vi "CRYCalibration Editor.vi"() -> ()   [LabVIEW 2013]
uses:
  <vilib>/Utility/miscctls.llb/LVBoundsTypeDef.ctl
  Typedef Control/CRYCalibration All Cluster.ctl
  Typedef Control/CRYCalibration 2DCluster.ctl
  Typedef Control/CRYCalibration Cluster.ctl
  Typedef Control/CRYData Cluster.ctl
  CRYProject/CRYProject Editor Global.vi
  CRYMainGlobal.vi
  CRYWindow/SubVI/CRYMain Sub Window Global.vi
  SubVI/CRYCal Global.vi
  Misc/SubVI/CRYMisc vis settings global.vi
panel:
  out "Signal Type Index":i32
  out "Origine Calibration":T1 {"Calibration 2D"."Sens Curve"."Z data" items=["dB", "Lin"]; "Calibration 2D"."Sens Curve"."X data" items=["dB", "Lin"]; "Calibration 2D"."Sens Curve"."Y data" items=["dB", "Lin"]; "Calibration 2D"."Sens Curve"."Z dB ref" format="%.1f"; "Calibration 2D"."Sens Curve"."Z axis" items=["Log", "Lin"]; "Calibration 2D"."Sens Curve"."X dB ref" format="%.1f"; "Calibration 2D"."Sens Curve"."X axis" items=["Log", "Lin"]; "Calibration 2D"."Sens Curve"."Y axis" items=["Log", "Lin"]; "Calibration 2D"."Sens Curve"."Y dB ref" format="%.1f"; "Calibration 2D"."Sens Curve"."Curve"."z" format="%.2f"; "Calibration 2D"."Sens Curve"."Curve"."y" format="%.2f"; "Calibration 2D"."Sens Curve"."Curve"."x" format="%.2f"; "Calibration 2D"."EQ Curve"."Z data" items=["dB", "Lin"]; "Calibration 2D"."EQ Curve"."X data" items=["dB", "Lin"]; "Calibration 2D"."EQ Curve"."Y data" items=["dB", "Lin"]; "Calibration 2D"."EQ Curve"."Z dB ref" format="%.1f"; "Calibration 2D"."EQ Curve"."Z axis" items=["Log", "Lin"]; "Calibration 2D"."EQ Curve"."X dB ref" format="%.1f"; "Calibration 2D"."EQ Curve"."X axis" items=["Log", "Lin"]; "Calibration 2D"."EQ Curve"."Y axis" items=["Log", "Lin"]; "Calibration 2D"."EQ Curve"."Y dB ref" format="%.1f"; "Calibration 2D"."EQ Curve"."Curve"."z" format="%.2f"; "Calibration 2D"."EQ Curve"."Curve"."y" format="%.2f"; "Calibration 2D"."EQ Curve"."Curve"."x" format="%.2f"; "Calibration 2D"."Corr Curve"."Z data" items=["dB", "Lin"]; "Calibration 2D"."Corr Curve"."X data" items=["dB", "Lin"]; "Calibration 2D"."Corr Curve"."Y data" items=["dB", "Lin"]; "Calibration 2D"."Corr Curve"."Z dB ref" format="%.1f"; "Calibration 2D"."Corr Curve"."Z axis" items=["Log", "Lin"]; "Calibration 2D"."Corr Curve"."X dB ref" format="%.1f"; "Calibration 2D"."Corr Curve"."X axis" items=["Log", "Lin"]; "Calibration 2D"."Corr Curve"."Y axis" items=["Log", "Lin"]; "Calibration 2D"."Corr Curve"."Y dB ref" format="%.1f"; "Calibration 2D"."Corr Curve"."Curve"."z" format="%.2f"; "Calibration 2D"."Corr Curve"."Curve"."y" format="%.2f"; "Calibration 2D"."Corr Curve"."Curve"."x" format="%.2f"; "Calibration 2D"."Calibration"."EQ Step size" items=["R10", "R20", "R40", "R80", "User"]; "Calibration 2D"."Calibration"."Corr Step size" items=["R10", "R20", "R40", "R80", "User"]}
  out "I_Calibrated Device Name":string[][](array[string])
  out "O_Calibrated Device Name":string[][](array[string])
  out "O_Signal Type Name":string[][](array[string])
  out "I_Signal Type Name":string[][](array[string])
  out "OuterEvent":bool
  out "Mode":string="Load"
  out "EndFlag":bool
  in  "AddStep":bool
  in  "Cal_ValueChange":bool
  out "Calibration":T1 {"Calibration 2D"."Sens Curve"."Z data" items=["dB", "Lin"]; "Calibration 2D"."Sens Curve"."X data" items=["dB", "Lin"]; "Calibration 2D"."Sens Curve"."Y data" items=["dB", "Lin"]; "Calibration 2D"."Sens Curve"."Z dB ref" format="%.1f"; "Calibration 2D"."Sens Curve"."Z axis" items=["Log", "Lin"]; "Calibration 2D"."Sens Curve"."X dB ref" format="%.1f"; "Calibration 2D"."Sens Curve"."X axis" items=["Log", "Lin"]; "Calibration 2D"."Sens Curve"."Y axis" items=["Log", "Lin"]; "Calibration 2D"."Sens Curve"."Y dB ref" format="%.1f"; "Calibration 2D"."Sens Curve"."Curve"."z" format="%.2f"; "Calibration 2D"."Sens Curve"."Curve"."y" format="%.2f"; "Calibration 2D"."Sens Curve"."Curve"."x" format="%.2f"; "Calibration 2D"."EQ Curve"."Z data" items=["dB", "Lin"]; "Calibration 2D"."EQ Curve"."X data" items=["dB", "Lin"]; "Calibration 2D"."EQ Curve"."Y data" items=["dB", "Lin"]; "Calibration 2D"."EQ Curve"."Z dB ref" format="%.1f"; "Calibration 2D"."EQ Curve"."Z axis" items=["Log", "Lin"]; "Calibration 2D"."EQ Curve"."X dB ref" format="%.1f"; "Calibration 2D"."EQ Curve"."X axis" items=["Log", "Lin"]; "Calibration 2D"."EQ Curve"."Y axis" items=["Log", "Lin"]; "Calibration 2D"."EQ Curve"."Y dB ref" format="%.1f"; "Calibration 2D"."EQ Curve"."Curve"."z" format="%.2f"; "Calibration 2D"."EQ Curve"."Curve"."y" format="%.2f"; "Calibration 2D"."EQ Curve"."Curve"."x" format="%.2f"; "Calibration 2D"."Corr Curve"."Z data" items=["dB", "Lin"]; "Calibration 2D"."Corr Curve"."X data" items=["dB", "Lin"]; "Calibration 2D"."Corr Curve"."Y data" items=["dB", "Lin"]; "Calibration 2D"."Corr Curve"."Z dB ref" format="%.1f"; "Calibration 2D"."Corr Curve"."Z axis" items=["Log", "Lin"]; "Calibration 2D"."Corr Curve"."X dB ref" format="%.1f"; "Calibration 2D"."Corr Curve"."X axis" items=["Log", "Lin"]; "Calibration 2D"."Corr Curve"."Y axis" items=["Log", "Lin"]; "Calibration 2D"."Corr Curve"."Y dB ref" format="%.1f"; "Calibration 2D"."Corr Curve"."Curve"."z" format="%.2f"; "Calibration 2D"."Corr Curve"."Curve"."y" format="%.2f"; "Calibration 2D"."Corr Curve"."Curve"."x" format="%.2f"; "Calibration 2D"."Calibration"."EQ Step size" items=["R10", "R20", "R40", "R80", "User"]; "Calibration 2D"."Calibration"."Corr Step size" items=["R10", "R20", "R40", "R80", "User"]}
  in  "Insert flag":bool
  in  "Setup in":string
  in  "Hardware In":string
  in  "Load Test":bool
  out "VIMiniumBound":T5
  out "Proper VI No":i32
  in  "Revert":bool
  in  "stop":bool
  in  "Board Tab":enum32{"Page 1", "Page 2"}(tab)
  in  "Cancel":bool caption="Apply"
  in  "SaveCalibration":bool caption="Apply"
  in  "Main Tab":enum32{"Input", "Output", "Help"}(tab)=enum."Output"
  in  "Input Signal Type":i32(ring) caption="输入信号通道" items=["Direct In 1", "Direct In 2", "Direct In 3", "Direct In 4", "Mic 1", "Mic 2", "Mic 3", "Mic 4", "DUT Mic L", "DUT Mic Current L", "Imp 1L", "Imp 1R", "LineIn L", "LineIn R", "USB In L", "USB In R"]
  out "6_In":bool
  in  "I_SCopy":bool caption="Open_Table"
  in  "I_SRename":bool caption="Open_Table"
  in  "I_SDelete":bool caption="Open_Table"
  in  "I_SAdd":bool caption="Open_Table"
  in  "Calibrated Input Device":i32(ring) caption="校准输入设备" items=["CRY33x Mic 1.dat", "CRY33x Mic 2.dat", "CRY33x Mic 3.dat", "CRY33x Mic 4.dat", "unity cal-in.dat", "USB In L.dat", "USB In R.dat"]
  in  "dB In":dbl caption="Sensitivity" format="%#.2g"
  out "3_In":bool
  out "2_In":bool
  in  "Calibrate In":bool caption="Calibrate"
  in  "CalibrationSeq In":u16(ring) caption="校准序列" items=["Mic Calibration"]
  out "dB ref In":dbl=1.0 caption="dB参考" format="%#_3p"
  out "unit In":string="V" caption="单位"
  in  "Units In":bool
  in  "Sensitivity In":dbl caption="灵敏度" format="%#_6p"
  in  "Channel In":i32(ring) caption="声卡通道" items=["Input 1", "Input 2", "Input 3", "Input 4"]
  out "Sens Value In":string caption="灵敏度值"
  out "Corre Curve In":string caption="修正曲线"
  out "1_In":bool
  out "Sens unit In":string="V/V"
  out "4_In":bool
  out "Input Channel Info":i32[](listbox)
  out "5_In":bool
  in  "I_Copy":bool caption="Open_Table"
  in  "I_Rename":bool caption="Open_Table"
  in  "I_Delete":bool caption="Open_Table"
  in  "I_Add":bool caption="Open_Table"
  in  "I_From CurveLib":bool caption="O_From CurveLib"
  in  "Hz In":dbl caption="Hz"
  in  "Hz Out":dbl caption="Hz"
  out "6_Out":bool
  in  "Output Signal Type":i32(ring) caption="输出信号通道" items=["Direct Out 1", "Direct Out 2", "Direct Out 3", "Direct Out 4", "Headphone 1L", "Headphone 1R", "Mouth Sim 1", "Mouth Sim 2", "USB Out L", "USB Out R"]
  in  "O_SCopy":bool caption="Open_Table"
  in  "O_SRename":bool caption="Open_Table"
  in  "O_SDelete":bool caption="Open_Table"
  in  "O_SAdd":bool caption="Open_Table"
  out "5_Out":bool
  out "Output Channel Info":i32[](listbox)
  out "4_Out":bool
  in  "dB Out":dbl caption="Sensitivity" format="%#.2g"
  in  "Channel Out":i32(ring) caption="声卡通道" items=["Output 1", "Output 2", "Output 3", "Output 4"]
  out "1_Out":bool
  out "Corre Curve Out":string caption="修正曲线"
  out "Sens Value Out":string caption="灵敏度值"
  in  "Sensitivity Out":dbl=1e-50 caption="灵敏度" min=1e-50 format="%#_6p"
  in  "Units Out":bool caption="Unit..."
  out "unit Out":string="V" caption="单位"
  out "dB ref Out":dbl=1.0 caption="dB参考" format="%#_3p"
  in  "CalibrationSeq Out":u16(ring) caption="校准序列" items=["Speaker Equalization 1", "Speaker Equalization 2"]
  in  "Calibrate Out":bool caption="Add"
  out "2_Out":bool
  out "3_Out":bool
  out "EQ Curve Out":string caption="均衡器曲线"
  out "Sens unit Out":string="V/V"
  in  "Calibrated Output Device":i32(ring) caption="校准输出设备" items=["CRY602 Mouth 1.dat", "CRY602 Mouth 2.dat", "unity cal-out.dat", "USB Out L.dat", "USB Out R.dat"]
  in  "O_Copy":bool caption="Open_Table"
  in  "O_Rename":bool caption="Open_Table"
  in  "O_Delete":bool caption="Open_Table"
  in  "O_Add":bool caption="Open_Table"
  in  "O_From CurveLib":bool
  in  "Help":string
  in  "Open_table":bool
  in  "Load...":bool caption="Apply"
  # "dB"
  # "dB"
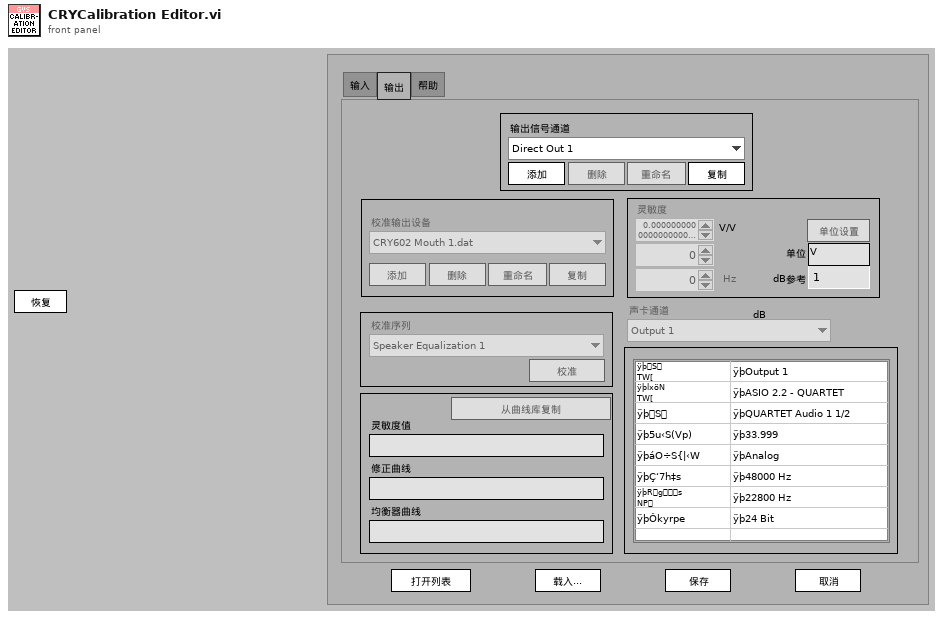
[diagram p1: front panel]
types:
  T1 = typedef "CRYCalibration All Cluster.ctl" = cluster{"Calibration 2D":T2[], "Help":string, "Tab Value":i32, "Input Signal Type":string, "Output Signal Type":string}
  T2 = typedef "CRYCalibration 2DCluster.ctl" = cluster{"Calibration":T3, "Corr Curve":T4, "EQ Curve":T4, "Sens Curve":T4}
  T3 = typedef "CRYCalibration Cluster.ctl" = cluster{"Calibration Step Name":string, "Device":string, "Correction Curve Name":string, "Equalization Curve Name":string, "Sensitivity Curve Name":string, "Corr Folder and File":string, "EQ Folder and File":string, "Sens Folder and File":string, "Corr Step size":u16, "EQ Step size":u16, "Input":bool, "Last Cal Date (sec)":timestamp, "Cha Name":string, "Corr Curve Found":bool, "EQ Curve Found":bool, "Sens Curve Found":bool, "Signal Type":string, "Calibrated Device":string, "Hz":u32}
  T4 = typedef "CRYData Cluster.ctl" = cluster{"Name":string, "Curve":cluster{"x":dbl, "y":dbl, "z":dbl}[], "X data":u16, "Y data":u16, "Z data":u16, "X axis":u16, "Y axis":u16, "Z axis":u16, "X unit":string, "Y unit":string, "Z unit":string, "X dB ref":dbl, "Y dB ref":dbl, "Z dB ref":dbl, "single val":bool, "protected":bool, "display X":bool, "display Y":bool, "display Z":bool, "Test Info":string, "Step No.":i32, "Plot Settings":cluster{"Color":u32, "Interpolation":u8, "Point Style":u8, "Line Style":u8, "Point Color":u32, "Line Width":u8, "Bar Plot Style":u8, "Fill To":i16}, "AutoProtect":bool}
  T5 = typedef "LVBoundsTypeDef.ctl" = cluster{"Width":u32, "Height":u32}
  T6 = typedef "CRYStep.ctl" = cluster{"No.VI":i32, "Category":string, "StepName":string, "Seq setup flattened":string, "Comment":string, "Steps config.":bool[], "Jump config":i32[], "Start":dbl, "Increment":dbl, "Name":string, "Unit":string, "Y data":u16, "Y prefix":string, "Y dB ref":dbl, "Y unit":string, "Repeat State Array":cluster{"Start":dbl, "Increment":dbl, "Count":i32, "Num":i32}[]}
  T7 = cluster{"Custom units dialog?":bool, "Use custom unit?":bool}
  T8 = enum16{"OK", "Yes", "YesNo", "YesNoCancel", "ReplaceAppend"}
  T9 = enum8{"Enabled", "Disabled", "Disabled and Grayed Out"}
  T10 = cluster{"Load Test":bool, "Units In":bool, "Calibrate In":bool, "Units Out":bool, "Calibrate Out":bool, "Open_table":bool, "Insert flag":bool, "Cal_ValueChange":bool, "I_Add":bool, "I_Delete":bool, "I_Rename":bool, "I_Copy":bool, "O_Add":bool, "O_Delete":bool, "O_Rename":bool, "O_Copy":bool, "I_SAdd":bool, "I_SDelete":bool, "I_SRename":bool, "I_SCopy":bool, "O_SAdd":bool, "O_SDelete":bool, "O_SRename":bool, "O_SCopy":bool, "I_From CurveLib":bool, "O_From CurveLib":bool, "SaveCalibration":bool, "Cancel":bool}
  T11 = typedef "CRYHardware.ctl" = cluster{"Name":string, "Analog I/O":u16, "Digital I/O":u16, "Channels":u8, "Dig Dev ID":u8, "N ports":u8, "Interface":u32, "Dig I/O Ports":cluster{"port #":i16, "width":i16, "direction":i32}[], "Interf settings":cluster{"Type":u16, "COM Port":u8, "Baud rate":u32, "Data bits":u32, "Parity":u16, "Stop bits":u16, "Flow control":u16, "Dev ID IEEE":u8}[], "N interfs":i32, "udev SNs":i16[], "udev enable":bool, "Channel Array":T12[], "Cal sequence":string, "SelectedIn":u16, "SelectedOut":u16, "SelectedTab":u16, "State":bool, "Help":string, "Advanced":bool, "In Audio Driver":u16, "Out Audio Driver":u16}
  T12 = typedef "CRYHardware Channel Info.ctl" = cluster{"ID":i32, "Name":string, "Digital":bool, "Input":bool, "Device Name":string, "Hardware Ch ID":u8, "Vmax (V)":dbl, "Latency (samples)":dbl, "Sampling Rate (Hz)":u32, "Bit Depth":u32, "Anti-aliasing Factor (%fs)":sgl, "DAQmx Channel":tag, "term config":i32, "Coupling":i32, "IEPE en":bool, "ASIOChannel Name":string, "Audio Driver":u16, "ASIOChannel Index":u8}
  T13 = cluster{"gen'r mode":i32, "frequency":u32, "output level":dbl, "wave path":string, "wav play mode":i32, "duration":dbl, "n times":i32, "channel":i32, "wav level":dbl, "EQ":bool, "f knob log":bool, "f knob low":dbl, "f knob high":dbl, "ol knob log":bool, "ol knob low":dbl, "ol knob high":dbl, "Lin Display Prefs":string, "dB Display Prefs":string, "Duration noise":dbl, "Min freq noise":dbl, "Max freq noise":dbl, "Signal Type":string, "Play Sine Wave":i32}
  T14 = cluster{"Calibrate":bool, "Calibrate":bool, "Calibrate":bool}
  T15 = typedef "CRYMultimeter.ctl" = cluster{"Ave/Max/Min":i32, "Level":i32, "Channel":i32, "Signal Type":string, "Weighting":string, "Applay Correction":bool, "lin/exp avg":u16, "rec time (sec)":dbl, "Average Time (Sec)":dbl, "Lin Display Prefs":string, "dB Display Prefs":string, "Time Weighting":u16, "Display":u16}
  T16 = cluster{"InputLevel":dbl, "unit":string, "dB ref.":dbl}
  T17 = typedef "CRYData Cluster Array.ctl" = T4[]
  T18 = typedef "CRYStimulus Cluster.ctl" = cluster{"StimulusType":string, "UseMLValArray":u16[], "ML_axisArray":u16[], "MLValLevelNameArray":string[], "Level(U)Array":dbl[], "Start(Stop)FreqArray":dbl[], "Start(Stop)AmpArray":dbl[], "StepResolutionArray":u16[], "Unit_Array":u16[], "DegValArray":dbl[], "DegUnitArray":string[], "Steps1":i32, "Cycle/step1(#)":u32, "Time/step1(s)":dbl, "Transition1":dbl, "SweepRate2":dbl, "Freq3(Hz)":dbl, "Steps3(#)":dbl, "Cycles3(#)":u32, "StepSize3":dbl, "wave time":string, "RMS_Value4":dbl, "Peak_Value4":dbl, "WavePath4":string, "RMS_unit4":string, "Peak_unit4":string, "wave Info":string, "dc_ctrl5_1":u16, "dc_ctrl5_2":u16, "dc_polar5":u16, "Max.Current":u16, "Steps5(#)":u32, "Time/Step5":dbl, "Level5":dbl, "StepsSize5Val":dbl, "StepSize5Unit":string, "SweepType":u16, "Fixed/Ratio6":u16, "Transition6":dbl, "Steps6(#)":dbl, "Cycle/Steps6(#)":u32, "Time/Steps6(s)":dbl, "Freq6(Hz)":dbl, "Difference6(Hz)":dbl, "Ratio6":string, "NoiseType7":u16, "Duration7(s)":dbl, "MinFreq7(Hz)":dbl, "MaxFreq7(Hz)":dbl, "MinFreq8(Hz)":dbl, "MaxFreq8(Hz)":dbl, "FreqRounding8":bool, "Duration8(s)":dbl, "Tones8":dbl, "RoundingVal8":dbl, "ApplyEQ":bool, "Duration(s)":dbl, "CustomStimulusName ":string, "Flatten Element Array":string[], "sine waves":cluster{"freq":dbl, "ampl":dbl, "cycles":dbl}[], "Channel Out":i32, "RatioVal6":dbl, "TabCtrl6":enum32{"Master Tone", "Slave Tone"}, "Signal Type Name":string, "Help":string, "Channel Sel":u16, "V on DUT":bool, "Output Imp":dbl, "Nominal Imp":dbl}
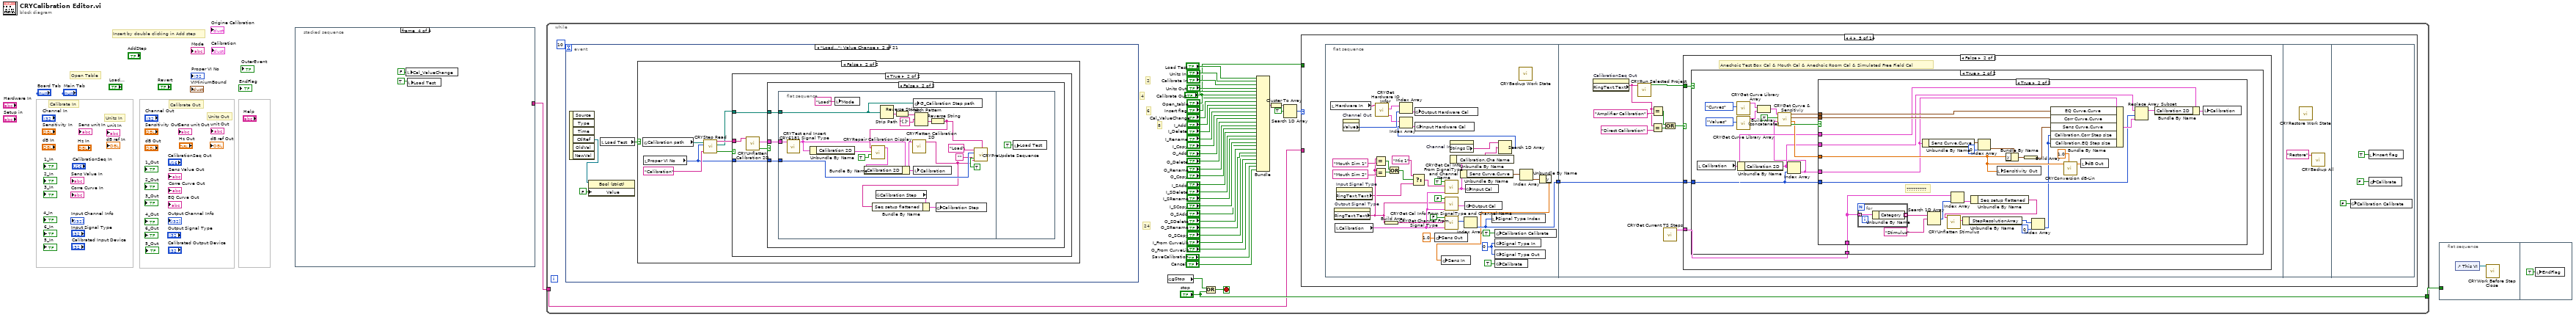
[diagram p0: block diagram]
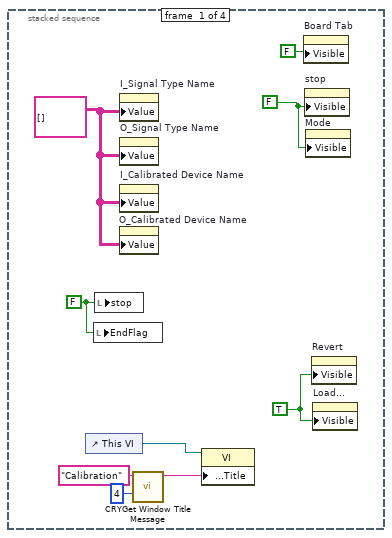
[diagram p2: hidden frame]
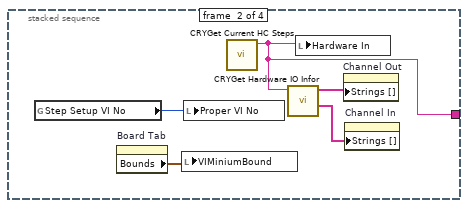
[diagram p3: hidden frame]
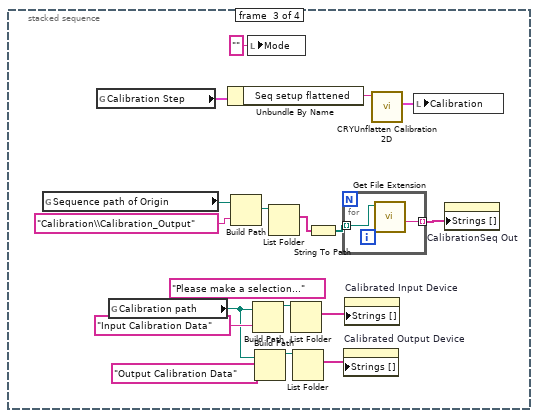
[diagram p4: hidden frame]
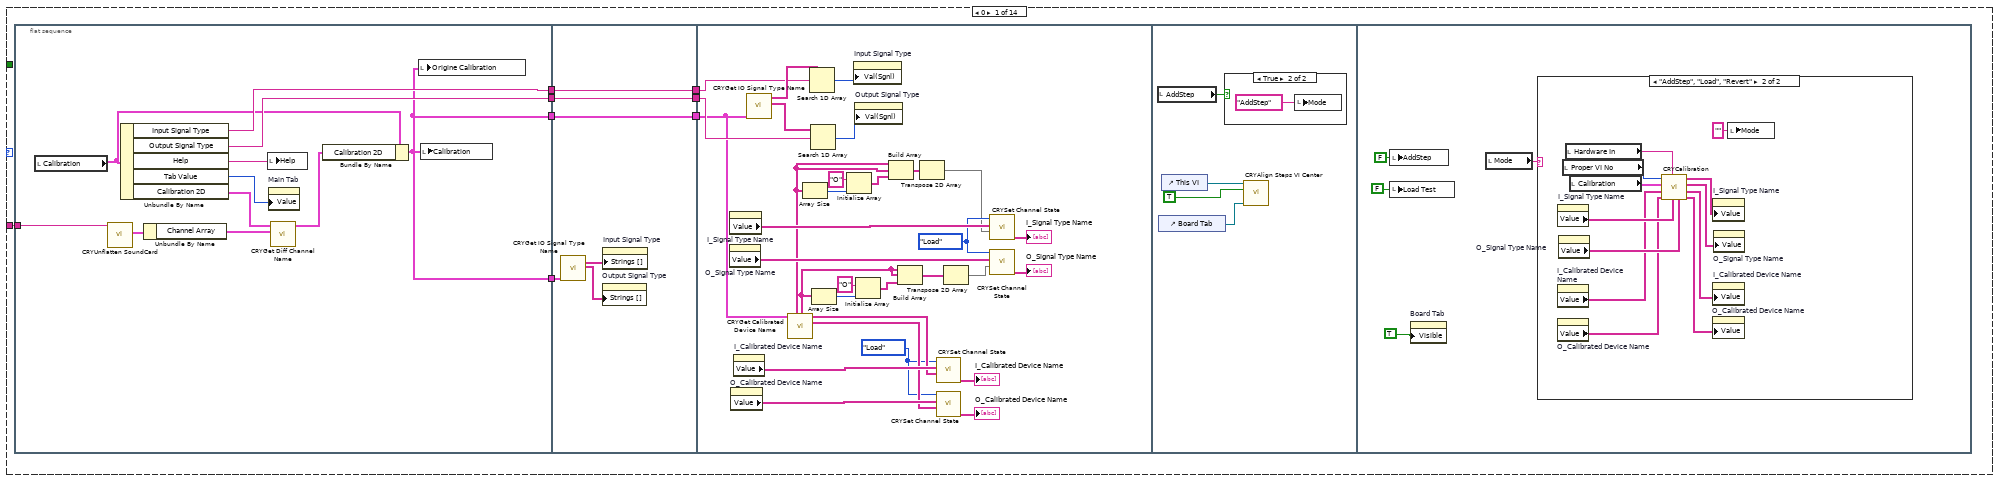
[diagram p5: hidden frame]
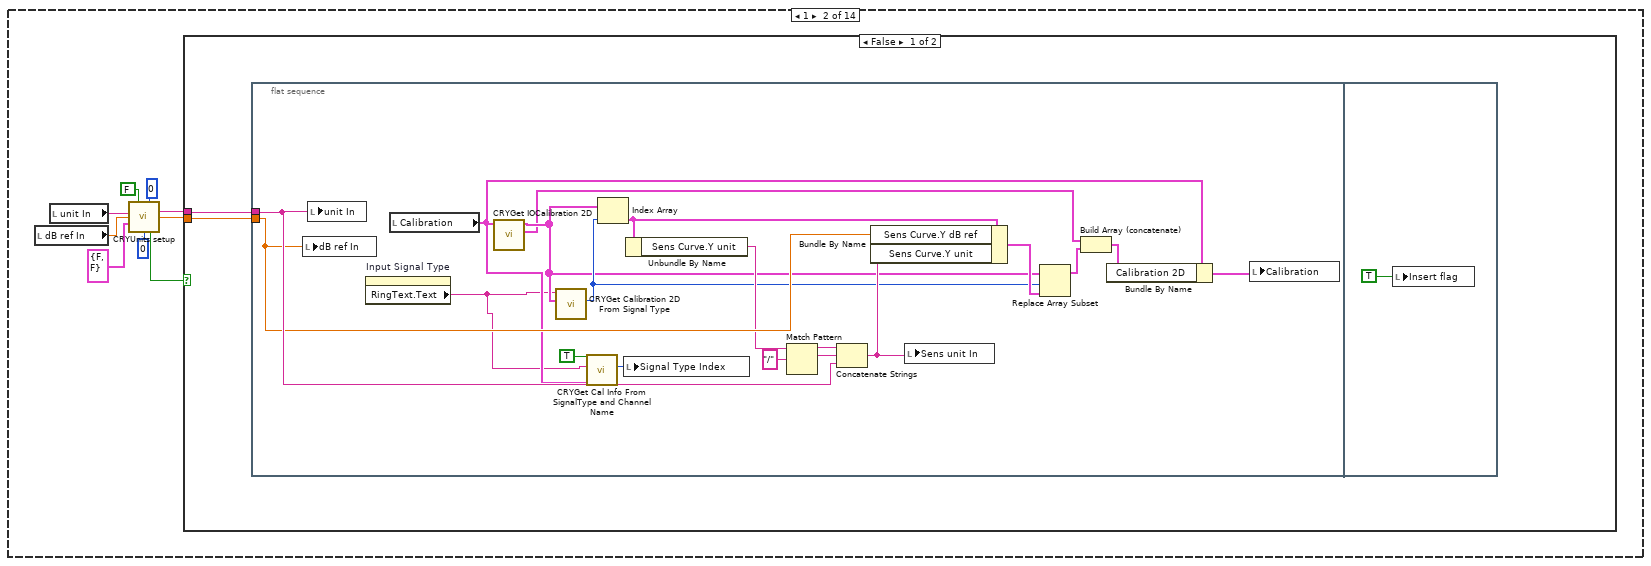
[diagram p8: hidden frame]
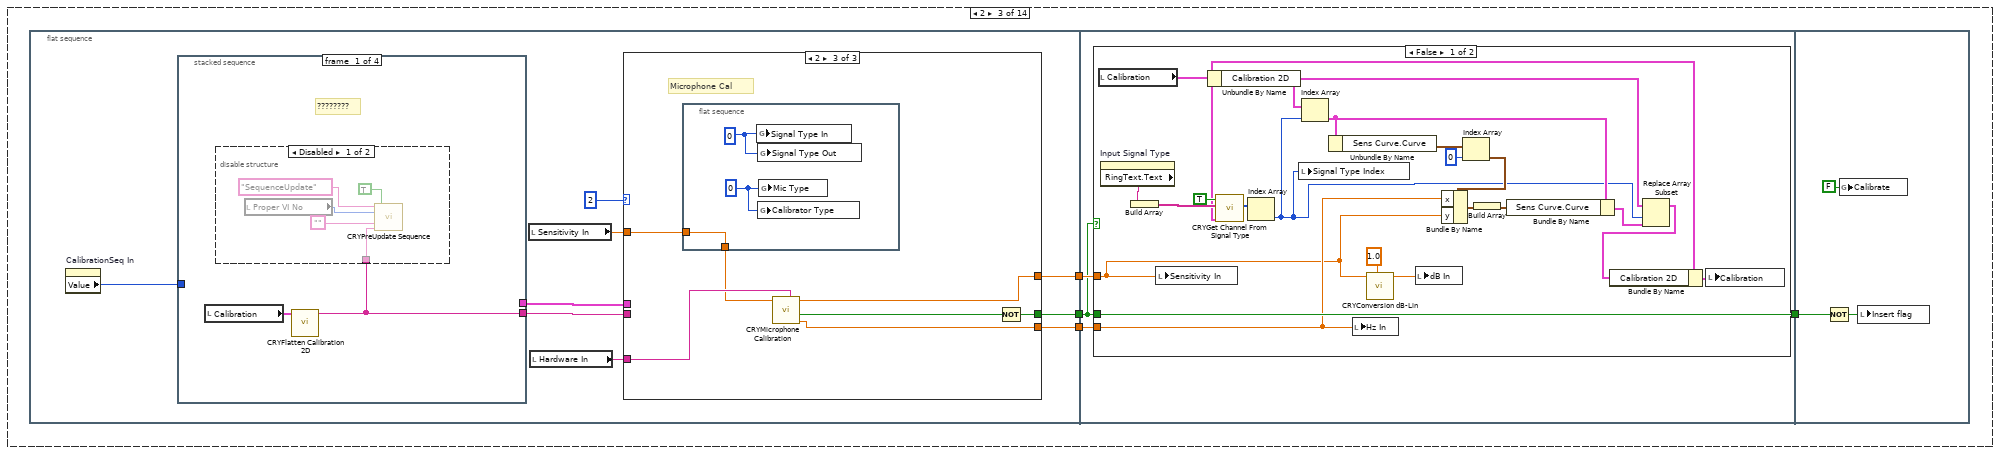
[diagram p10: hidden frame]
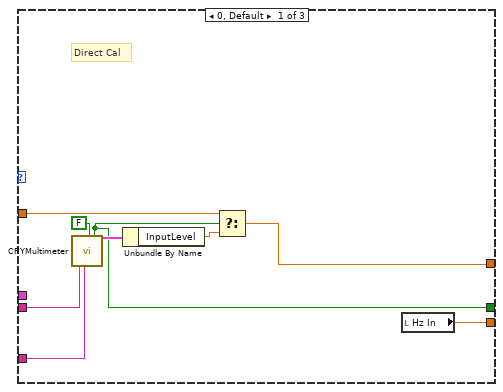
[diagram p11: hidden frame]
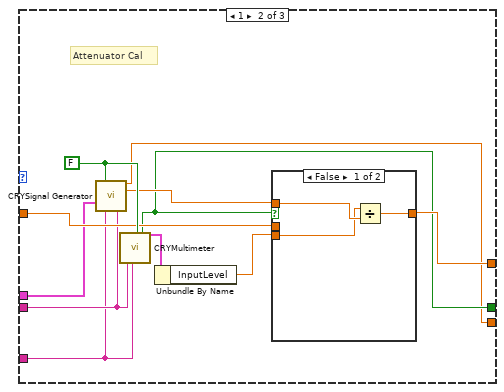
[diagram p12: hidden frame]
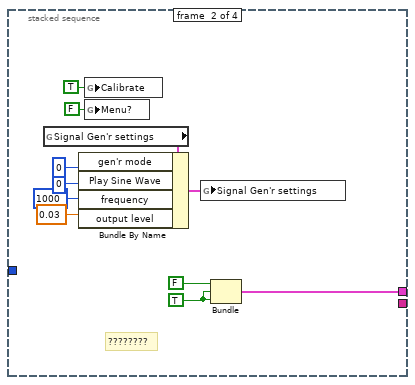
[diagram p15: hidden frame]
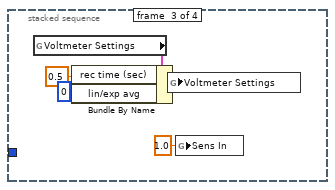
[diagram p16: hidden frame]
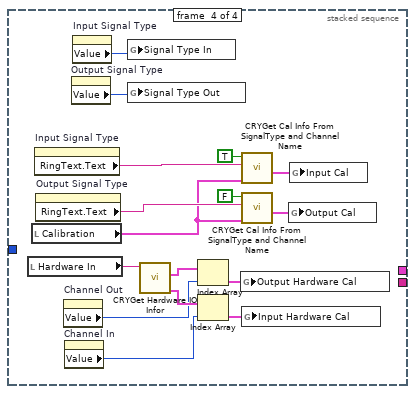
[diagram p17: hidden frame]
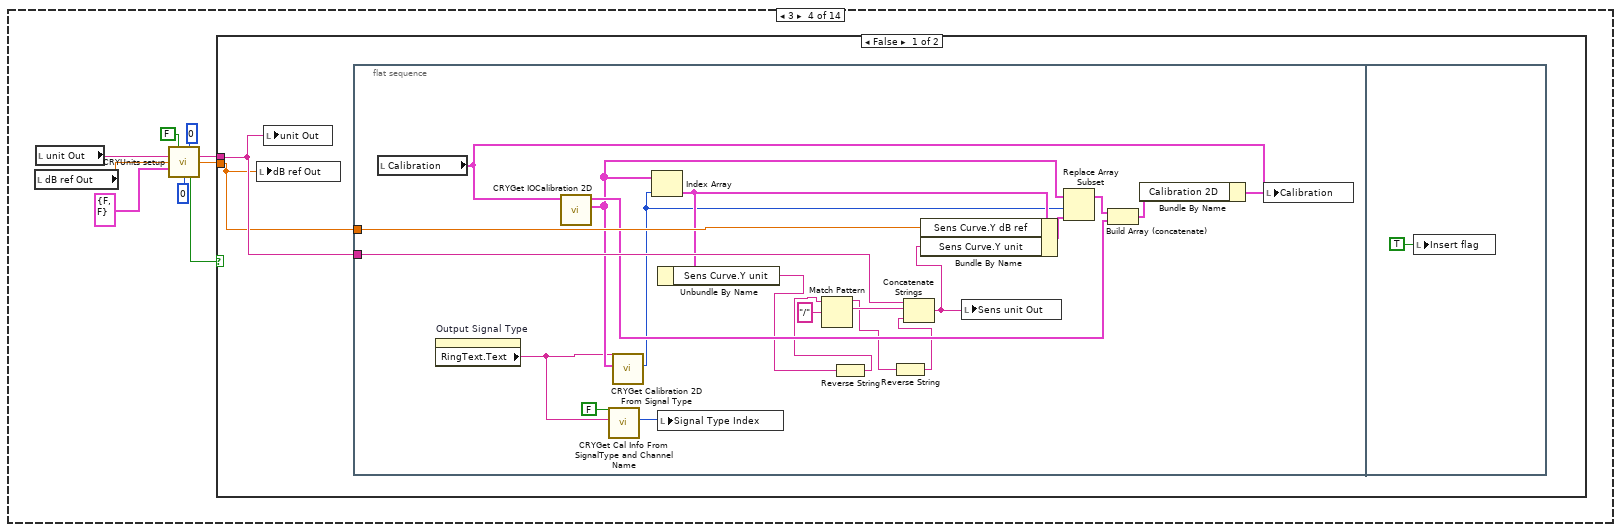
[diagram p19: hidden frame]
diagram:
  # "Insert by double clicking in Add step"
  # "Calibrate Out"
  # "Calibrate In"
  # "Units Out"
  # "Units In"
  # "Open Table"
  n1 = stacked-sequence {
    tunnel: [_ w12 _ _] -> w2
    frame #0 {
      w8 = TRUE ("Visible")
      w7 = FALSE ("Visible")
      w10 = string[][] [] ("I_Name")
      w11 = FALSE ("Data View Auto Open?")
      n2 = control-ref of="This VI"() -> (w3:refnum<vi>)
      n3 = local write "EndFlag"(w11) -> ()
      n4 = local write "stop"(w11) -> ()
      n5 = property on="I_Signal Type Name" class="Arr (strict)"("Value"=w10) -> ()  [unwired: 2 in, 2 out]
      n6 = property on="O_Signal Type Name" class="Arr (strict)"("Value"=w10) -> ()  [unwired: 2 in, 2 out]
      n7 = property on="I_Calibrated Device Name" class="Arr (strict)"("Value"=w10) -> ()  [unwired: 2 in, 2 out]
      n8 = property on="O_Calibrated Device Name" class="Arr (strict)"("Value"=w10) -> ()  [unwired: 2 in, 2 out]
      n9 = call "CRYGet Window Title Message.vi"("No"=4, "Kind"="Calibration") -> ("Multibyte String"=w4:string)  [unwired: 4 in, 5 out]
      n10 = property class="VI"(reference=w3, "Front Panel.Title"=w4) -> ()  [unwired: 1 in, 2 out]
      n11 = property on="Board Tab" class="TabCtl (strict)"("Visible"=FALSE) -> ()  [unwired: 2 in, 2 out]
      n12 = property on="stop" class="Bool (strict)"("Visible"=w7) -> ()  [unwired: 2 in, 2 out]
      n13 = property on="Mode" class="Str"("Visible"=w7) -> ()  [unwired: 2 in, 2 out]
      n14 = property on="Revert" class="Bool (strict)"("Visible"=w8) -> ()  [unwired: 2 in, 2 out]
      n15 = property on="Load..." class="Bool (strict)"("Visible"=w8) -> ()  [unwired: 2 in, 2 out]
    }
    frame #1 {
      n16 = global read "CRYProject Editor Global.vi" "Step Setup VI No"() -> (w14:i32)
      n17 = property on="Board Tab" class="TabCtl (strict)"() -> ("Bounds"=w13:T5)  [unwired: 2 in, 2 out]
      n18 = local write "VIMiniumBound"(w13) -> ()
      n19 = local write "Proper VI No"(w14) -> ()
      n20 = call "CRYGet Current HC Steps.vi"() -> ("Hardware setup flattened Out"=w12:string)  [unwired: 10 in, 1 out]
      n21 = call "CRYGet Hardware IO Infor.vi"("Hardware setup In"=w12) -> ("I_Hardware Channel Name Out"=w15:string[], "O_Hardware Channel Name Out"=w16:string[])  [unwired: 9 out]
      n22 = local write "Hardware In"(w12) -> ()
      n23 = property on="Channel Out" class="Ring (strict)"("Strings []"=w16) -> ()  [unwired: 2 in, 2 out]
      n24 = property on="Channel In" class="Ring (strict)"("Strings []"=w15) -> ()  [unwired: 2 in, 2 out]
    }
    frame #2 {
      (unwired) "Please make a selection..."
      n25 = global read "CRYMainGlobal.vi" "Sequence path of Origin"() -> (w17:path)
      n26 = global read "CRYProject Editor Global.vi" "Calibration Step"() -> (w21:T6)
      n27 = global read "CRYMainGlobal.vi" "Calibration path"() -> (w29:path)
      n28 = Unbundle By Name(w21) -> ("Seq setup flattened"=w20:string)
      n29 = Build Path(base path=w17, name or relative path="Calibration\\Calibration_Output") -> (appended path=w24:path)
      n30 = local write "Mode"("" ("reversed")) -> ()
      n31 = Build Path(base path=w29, name or relative path="Input Calibration Data") -> (appended path=w32:path)
      n32 = Build Path(base path=w29, name or relative path="Output Calibration Data") -> (appended path=w31:path)
      n33 = List Folder(path=w24) -> (filenames=w23:string[])  [unwired: 3 in, 3 out]
      n34 = List Folder(path=w32) -> (filenames=w28:string[])  [unwired: 3 in, 3 out]
      n35 = List Folder(path=w31) -> (filenames=w27:string[])  [unwired: 3 in, 3 out]
      n36 = String To Path(string=w23) -> (path=w22:path[])
      n37 = for {
        tunnel: w22 -> [w35] mode=indexing
        tunnel: [w34] -> w25 mode=indexing
        n38 = call <vilib>:"Get File Extension.vi"("file"=w35) -> ("filename without extension"=w34:string)  [unwired: 7 in, 3 out]
      }
      n39 = property on="Calibrated Output Device" class="Ring (strict)"("Strings []"=w27) -> ()  [unwired: 2 in, 2 out]
      n40 = property on="Calibrated Input Device" class="Ring (strict)"("Strings []"=w28) -> ()  [unwired: 2 in, 2 out]
      n41 = call "CRYUnflatten Calibration 2D.vi"("Flattened Calibration"=w20) -> ("Calibration Step Out"=w18:T1)  [unwired: 2 in, 8 out]
      n42 = local write "Calibration"(w18) -> ()
      n43 = property on="CalibrationSeq Out" class="Ring (strict)"("Strings []"=w25) -> ()  [unwired: 2 in, 2 out]
    }
    frame #3 {
      n44 = local write "Cal_ValueChange"(FALSE ("Cal_ValueChange")) -> ()
      n45 = local write "Load Test"(TRUE ("Load Test")) -> ()
    }
  }
  n46 = while {
    tunnel: w2 -> [w40]
    tunnel: ["stop"] -> w1
    stop <- w62 stop-if-true
    # "6"
    # "24"
    # "4"
    # "2"
    # "8"
    n47 = event shown="[1] \"Load...\": Value Change" {
      selector: _ -> [_ _ _ _ _ _ _ _ _ _ _ _ _ _ _ _ _ _ _ _ _]
      dyn-events: _ -> [_ _ _ _ _ _ _ _ _ _ _ _ _ _ _ _ _ _ _ _ _]
      timeout: 10 -> [_ _ _ _ _ _ _ _ _ _ _ _ _ _ _ _ _ _ _ _ _]
      event Timeout {
        n48 = event-data() -> ()  [unwired: 3 out]
      }
      event "Load...": Value Change {
        n49 = event-data() -> ("CtlRef"=w966:refnum<vi>)  [unwired: 6 out]
        n50 = property class="Bool (strict)"(reference=w966, "Value"=FALSE) -> ()  [unwired: 1 in, 2 out]
        n51 = local read "Load Test"() -> (w968:bool)
        n52 = case shown="False" w968 {
          frame True {
          }
          frame False {
            n53 = global read "CRYMainGlobal.vi" "Calibration path"() -> (w971:path)
            n54 = local read "Proper VI No"() -> (w969:i32)
            n55 = call "CRYStep Read.vi"("Category Name"="Calibration" ("Step File Name"), "Proper VI No"=w969, "Step File Path"=w971) -> ("status"=w972:bool, "selected path"=w970:path, "Flatten Step"=w973:string)  [unwired: 1 in, 3 out]
            n56 = case shown="True" w972 {
              tunnel: w973 -> [_ w977]
              tunnel: w970 -> [_ w978]
              tunnel: w969 -> [_ w975]
              frame False {
              }
              frame True {
                n57 = call "CRYUnflatten Calibration 2D.vi"("Flattened Calibration"=w977) -> ("Error?"=w979:bool, "Calibration Step Out"=w976:T1)  [unwired: 2 in, 7 out]
                n58 = case shown="False" w979 {
                  tunnel: w978 -> [_ w982]
                  tunnel: w976 -> [_ w981]
                  tunnel: w975 -> [_ w980]
                  frame True {
                  }
                  frame False {
                    n59 = flat-sequence {
                      tunnel: w982 -> [w985]
                      tunnel: w981 -> [w984]
                      tunnel: w980 -> [w995]
                      frame #0 {
                        n60 = call "CRYTest and Insert CRY6181 Signal Type.vi"("Calibration In"=w984) -> ("Calibration out"=w983:T1)  [unwired: 9 in, 1 out]
                        n61 = Unbundle By Name(w983) -> ("Calibration 2D"=w998:T2[])
                        n62 = local write "Mode"("Load" ("reversed")) -> ()
                        n63 = global read "CRYProject Editor Global.vi" "Calibration Step"() -> (w988:T6)
                        n64 = Strip Path(path=w985) -> (name=w999:string)  [unwired: 1 out]
                        n65 = Reverse String(1:w999) -> (0:w1001:string)
                        n66 = global write "CRYProject Editor Global.vi" "G_Calibration Step path"(w985) -> ()
                        n67 = Match Pattern(string=w1001, regular expression="[.]") -> (after substring=w1002:string)  [unwired: 4 out]
                        n68 = Reverse String(1:w1002) -> (0:w994:string)
                        n69 = call "CRYRepair Calibration Display.vi"("Calibration.Last Ch Changing?"=TRUE, "Calibration In"=w998, "Calibration Step Name"=w994) -> ("Calibration Out"=w997:T2[])  [unwired: 8 out]
                        n70 = Bundle By Name(cluster=w983, "Calibration 2D"=w997) -> (w992:T1)
                        n71 = call "CRYFlatten Calibration 2D.vi"("Calibration All Cluster"=w992) -> ("Calibration flattened"=w986:string)  [unwired: 10 in]
                        n72 = Bundle By Name(cluster=w988, "Seq setup flattened"=w986) -> (w987:T6)
                        n73 = local write "Calibration"(w992) -> ()
                        n74 = global write "CRYProject Editor Global.vi" "Calibration Step"(w987) -> ()
                        n75 = call "CRYPreUpdate Sequence.vi"("EventName"="Load", "StepName Arg3"=w994, "Proper VI No"=w995, "Project View Step Name Identifier Arg1"="", "Step flattened Arg2"=w986, "AllChangeFlg"=TRUE ("Name/Identifier")) -> ()  [unwired: 10 in]
                      }
                      frame #1 {
                        n76 = local write "Load Test"(TRUE ("Load Test")) -> ()
                      }
                    }
                  }
                }
              }
            }
          }
        }
      }
      event "Revert": Value Change {
        n77 = event-data() -> ("CtlRef"=w1005:refnum<vi>)  [unwired: 6 out]
        n78 = flat-sequence {
          frame #0 {
            # "Update????"
            n79 = global read "CRYProject Editor Global.vi" "Calibration Step"() -> (w1008:T6)
            n80 = Unbundle By Name(w1008) -> ("StepName"=w1007:string, "Seq setup flattened"=w1006:string)
            n81 = call "CRYUnflatten Calibration 2D.vi"("Flattened Calibration"=w1006) -> ("Calibration Step Out"=w1009:T1)  [unwired: 2 in, 8 out]
            n82 = Unbundle By Name(w1009) -> ("Calibration 2D"=w1013:T2[])
            n83 = call "CRYRepair Calibration Display.vi"("Calibration.Last Ch Changing?"=TRUE, "Calibration In"=w1013, "Calibration Step Name"=w1007) -> ("Calibration Out"=w1012:T2[])  [unwired: 8 out]
            n84 = Bundle By Name(cluster=w1009, "Calibration 2D"=w1012) -> (w1011:T1)
            n85 = disable-structure shown="Disabled" {
              frame Disabled {
                n86 = local write "Mode"("Revert" ("reversed")) -> ()
              }
              frame Enabled {
              }
            }
            n87 = local write "Calibration"(w1011) -> ()
          }
          frame #1 {
            n88 = local write "Load Test"(TRUE ("Load Test")) -> ()
          }
        }
        n89 = property class="Bool (strict)"(reference=w1005, "Value"=FALSE) -> ()  [unwired: 1 in, 2 out]
      }
      event Panel Close {
        n90 = event-data() -> ()  [unwired: 5 out]
        n91 = control-ref of="This VI"() -> (w1017:refnum<vi>)
        n92 = local write "Cancel"(TRUE ("Cancel")) -> ()
        n93 = call "CRYWork Before Step Close.vi"("StepVI Ref"=w1017) -> ()  [unwired: 11 in]
      }
      event "Input Signal Type": Value Change {
        n94 = event-data() -> ()  [unwired: 7 out]
        n95 = local read "Calibration"() -> (w1026:T1)
        n96 = property on="Input Signal Type" class="Ring (strict)"() -> ("RingText.Text"=w1022:string)  [unwired: 2 in, 2 out]
        n97 = Unbundle By Name(w1026) -> ("Calibration 2D"=w1037:T2[])
        n98 = call "CRYGet Button State Calibration.vi"("Signal Type Name"=w1022, "Input/Output"=TRUE) -> ("Mic or MouseSim State"=w1018:T9, "State"=w1020:T9)  [unwired: 5 in, 3 out]
        n99 = call "CRYGet Cal Info From SignalType and Channel Name.vi"("Calibration"=w1026, "Signal Type"=w1022, "In/Out?"=TRUE) -> ("Index"=w1023:i32)  [unwired: 6 in, 2 out]
        n100 = property on="I_SDelete" class="Bool"("DisabledEnum"=w1020) -> ()  [unwired: 2 in, 2 out]
        n101 = property on="I_Add" class="Bool"("DisabledEnum"=w1018) -> ()  [unwired: 2 in, 2 out]
        n102 = property on="I_Copy" class="Bool"("DisabledEnum"=w1018) -> ()  [unwired: 2 in, 2 out]
        n103 = property on="Calibrated Input Device" class="Ring (strict)"("DisabledEnum"=w1018) -> ()  [unwired: 2 in, 2 out]
        n104 = property on="I_SRename" class="Bool"("DisabledEnum"=w1020) -> ()  [unwired: 2 in, 2 out]
        n105 = Bundle By Name(cluster=w1026, "Input Signal Type"=w1022) -> (w1027:T1)
        n106 = Index Array(array=w1037, index=w1023) -> (element=w1036:T2)
        n107 = Unbundle By Name(w1036) -> ("Calibration.Calibrated Device"=w1024:string, "Calibration.Cha Name"=w1032:string, "Calibration.Device"=w1025:string)
        n108 = property on="Sensitivity In" class="DigNum (strict)"("DisabledEnum"=w1020) -> ()  [unwired: 2 in, 2 out]
        n109 = property on="dB In" class="DigNum (strict)"("DisabledEnum"=w1020) -> ()  [unwired: 2 in, 2 out]
        n110 = property on="Hz In" class="DigNum (strict)"("DisabledEnum"=w1020) -> ()  [unwired: 2 in, 2 out]
        n111 = property on="Units In" class="Bool"("DisabledEnum"=w1020) -> ()  [unwired: 2 in, 2 out]
        n112 = local write "Calibration"(w1027) -> ()
        n113 = property on="Channel In" class="Ring (strict)"("DisabledEnum"=w1020) -> ()  [unwired: 2 in, 2 out]
        n114 = property on="Calibrate In" class="Bool"("DisabledEnum"=w1020) -> ()  [unwired: 2 in, 2 out]
        n115 = property on="I_From CurveLib" class="Bool"("DisabledEnum"=w1020) -> ()  [unwired: 2 in, 2 out]
        n116 = property on="Channel In" class="Ring (strict)"() -> ("Strings []"=w1033:string[])  [unwired: 2 in, 2 out]
        n117 = property on="Calibrated Input Device" class="Ring (strict)"() -> ("Strings []"=w1035:string[])  [unwired: 2 in, 2 out]
        n118 = property on="CalibrationSeq In" class="Ring (strict)"() -> ("Strings []"=w1029:string[])  [unwired: 2 in, 2 out]
        n119 = Search 1D Array(1D array=w1033, element=w1032) -> (index of element=w1031:i32)  [unwired: 1 in]
        n120 = Search 1D Array(1D array=w1035, element=w1024) -> (index of element=w1034:i32)  [unwired: 1 in]
        n121 = Search 1D Array(1D array=w1029, element=w1025) -> (index of element=w1030:i32)  [unwired: 1 in]
        n122 = property on="Channel In" class="Ring (strict)"("Val(Sgnl)"=w1031) -> ()  [unwired: 2 in, 2 out]
        n123 = case shown="-1, Default" w1030 {
          tunnel: w1030 -> [w1039 _]
          tunnel: [w1039 0 ("index of element")] -> w1028
          frame 0 {
          }
          frame -1, Default {
          }
        }
        n124 = case shown="0, Default" w1034 {
          tunnel: w1034 -> [w1041 _]
          tunnel: [w1041 0 ("index of element")] -> w1019
          frame 0, Default {
          }
          frame -1 {
          }
        }
        n125 = property on="Calibrated Input Device" class="Ring (strict)"("Val(Sgnl)"=w1019) -> ()  [unwired: 2 in, 2 out]
        n126 = property on="CalibrationSeq In" class="Ring (strict)"("Value"=w1028) -> ()  [unwired: 2 in, 2 out]
      }
      event "Output Signal Type": Value Change {
        n127 = event-data() -> ()  [unwired: 7 out]
        n128 = local read "Calibration"() -> (w1051:T1)
        n129 = property on="Output Signal Type" class="Ring (strict)"() -> ("RingText.Text"=w1049:string)  [unwired: 2 in, 2 out]
        n130 = call "CRYGet Button State Calibration.vi"("Signal Type Name"=w1049, "Input/Output"=FALSE) -> ("Mouth Sim"=w1044:bool, "Mic or MouseSim State"=w1045:T9, "State"=w1047:T9, "Mouth Sim Number"=w1043:i32)  [unwired: 5 in, 1 out]
        n131 = Unbundle By Name(w1051) -> ("Calibration 2D"=w1064:T2[])
        n132 = call "CRYGet Cal Info From SignalType and Channel Name.vi"("Calibration"=w1051, "Signal Type"=w1049, "In/Out?"=FALSE) -> ("Index"=w1063:i32)  [unwired: 6 in, 2 out]
        n133 = property on="O_SDelete" class="Bool"("DisabledEnum"=w1047) -> ()  [unwired: 2 in, 2 out]
        n134 = property on="O_SRename" class="Bool"("DisabledEnum"=w1047) -> ()  [unwired: 2 in, 2 out]
        n135 = property on="O_Add" class="Bool"("DisabledEnum"=w1045) -> ()  [unwired: 2 in, 2 out]
        n136 = property on="O_Copy" class="Bool"("DisabledEnum"=w1045) -> ()  [unwired: 2 in, 2 out]
        n137 = property on="Calibrated Output Device" class="Ring (strict)"("DisabledEnum"=w1045) -> ()  [unwired: 2 in, 2 out]
        n138 = Index Array(array=w1064, index=w1063) -> (element=w1062:T2)
        n139 = Unbundle By Name(w1062) -> ("Calibration.Calibrated Device"=w1060:string, "Calibration.Cha Name"=w1056:string, "Calibration.Device"=w1052:string)
        n140 = Bundle By Name(cluster=w1051, "Output Signal Type"=w1049) -> (w1050:T1)
        n141 = property on="Sensitivity Out" class="DigNum (strict)"("DisabledEnum"=w1047) -> ()  [unwired: 2 in, 2 out]
        n142 = property on="dB Out" class="DigNum (strict)"("DisabledEnum"=w1047) -> ()  [unwired: 2 in, 2 out]
        n143 = property on="Hz Out" class="DigNum (strict)"("DisabledEnum"=w1047) -> ()  [unwired: 2 in, 2 out]
        n144 = property on="Units Out" class="Bool"("DisabledEnum"=w1047) -> ()  [unwired: 2 in, 2 out]
        n145 = local write "Calibration"(w1050) -> ()
        n146 = property on="O_From CurveLib" class="Bool"("DisabledEnum"=w1047) -> ()  [unwired: 2 in, 2 out]
        n147 = property on="Channel Out" class="Ring (strict)"("DisabledEnum"=w1047) -> ()  [unwired: 2 in, 2 out]
        n148 = property on="Calibrate Out" class="Bool"("DisabledEnum"=w1047) -> ()  [unwired: 2 in, 2 out]
        n149 = property on="CalibrationSeq Out" class="Ring (strict)"() -> ("Strings []"=w1054:string[])  [unwired: 2 in, 2 out]
        n150 = property on="Channel Out" class="Ring (strict)"() -> ("Strings []"=w1058:string[])  [unwired: 2 in, 2 out]
        n151 = property on="Calibrated Output Device" class="Ring (strict)"() -> ("Strings []"=w1061:string[])  [unwired: 2 in, 2 out]
        n152 = Search 1D Array(1D array=w1058, element=w1056) -> (index of element=w1057:i32)  [unwired: 1 in]
        n153 = Search 1D Array(1D array=w1054, element=w1052) -> (index of element=w1055:i32)  [unwired: 1 in]
        n154 = Search 1D Array(1D array=w1061, element=w1060) -> (index of element=w1059:i32)  [unwired: 1 in]
        n155 = property on="Channel Out" class="Ring (strict)"("Val(Sgnl)"=w1057) -> ()  [unwired: 2 in, 2 out]
        n156 = case shown="0, Default" w1059 {
          tunnel: w1059 -> [w1066 _]
          tunnel: [w1066 0 ("index of element")] -> w1046
          frame 0, Default {
          }
          frame -1 {
          }
        }
        n157 = case shown="False" w1044 {
          tunnel: w1055 -> [w1069 _]
          tunnel: [w1068 w1072] -> w1053
          tunnel: w1043 -> [_ w1072]
          frame False {
            n158 = case shown="-1, Default" w1069 {
              tunnel: w1069 -> [w1070 _]
              tunnel: [w1070 0 ("index of element")] -> w1068
              frame 0 {
              }
              frame -1, Default {
              }
            }
          }
          frame True {
          }
        }
        n159 = property on="Calibrated Output Device" class="Ring (strict)"("Val(Sgnl)"=w1046) -> ()  [unwired: 2 in, 2 out]
        n160 = property on="CalibrationSeq Out" class="Ring (strict)"("Value"=w1053) -> ()  [unwired: 2 in, 2 out]
      }
      event "Calibrated Input Device": Value Change {
        n161 = event-data() -> ()  [unwired: 7 out]
        n162 = local read "Origine Calibration"() -> (w1082:T1)
        n163 = property on="Input Signal Type" class="Ring (strict)"() -> ("RingText.Text"=w1075:string)  [unwired: 2 in, 2 out]
        n164 = local read "Calibration"() -> (w1073:T1)
        n165 = property on="Calibrated Input Device" class="Ring (strict)"() -> ("RingText.Text"=w1077:string)  [unwired: 2 in, 2 out]
        n166 = call "CRYGet Cal Info From SignalType and Channel Name.vi"("Calibration"=w1073, "Signal Type"=w1075, "In/Out?"=TRUE) -> ("Calibration 2D Cluster"=w1078:T2)  [unwired: 6 in, 2 out]
        n167 = Unbundle By Name(w1078) -> ("Calibration.Calibrated Device"=w1076:string)
        n168 = Equal?(x=w1077, y="unity cal-in.dat") -> (x = y?=w1086:bool)
        n169 = call "CRYTest Changing State.vi"("Origine Calibration"=w1082, "New Calibration"=w1073, "Signal Type"=w1075, "In/Out?"=TRUE) -> ("Changed/Added"=w1080:bool)  [unwired: 5 in, 2 out]
        n170 = Select(t=T9."Disabled and Grayed Out" ("Disabled"), s=w1086, f=T9."Enabled" ("Disabled")) -> (s? t:f=w1084:T9)
        n171 = Equal?(x=w1077, y=w1076) -> (x = y?=w1074:bool)
        n172 = property on="I_Delete" class="Bool"("DisabledEnum"=w1084) -> ()  [unwired: 2 in, 2 out]
        n173 = property on="I_Rename" class="Bool"("DisabledEnum"=w1084) -> ()  [unwired: 2 in, 2 out]
        n174 = property on="Sensitivity In" class="DigNum (strict)"("DisabledEnum"=w1084) -> ()  [unwired: 2 in, 2 out]
        n175 = And(x=w1080, y=w1074) -> (x .and. y?=w1079:bool)
        n176 = property on="Hz In" class="DigNum (strict)"("DisabledEnum"=w1084) -> ()  [unwired: 2 in, 2 out]
        n177 = property on="dB In" class="DigNum (strict)"("DisabledEnum"=w1084) -> ()  [unwired: 2 in, 2 out]
        n178 = case shown="False" w1079 {
          tunnel: w1077 -> [w1089 w1134]
          tunnel: w1075 -> [_ w1135]
          frame False {
            n179 = global read "CRYMainGlobal.vi" "Calibration path"() -> (w1095:path)
            n180 = Concatenate Strings("Input Calibration Data" ("name or relative path"), "\\" ("string"), w1089) -> (w1091:string)
            n181 = Build Path(base path=w1095, name or relative path=w1091) -> (appended path=w1094:path)
            n182 = call "CRYFlatten Data Read.vi"("Path In"=w1094) -> ("error out"=w1090:errorcluster, "Flatten Data Out"=w1096:string)  [unwired: 6 in, 1 out]
            n183 = case shown="No Error" w1090 {
              tunnel: w1096 -> [w1131 _]
              tunnel: w1089 -> [w1102 _]
              frame No Error {
                n184 = local read "Calibration"() -> (w1119:T1)
                n185 = call "CRYUnflatten Calibration Data File.vi"("Flattened Calibration"=w1131) -> ("Calibration 2D Data File Out"=w1130:T2)  [unwired: 8 in, 2 out]
                n186 = property on="Input Signal Type" class="Ring (strict)"() -> ("RingText.Text"=w1120:string)  [unwired: 2 in, 2 out]
                n187 = Unbundle By Name(w1130) -> ("Corr Curve"=w1124:T4, "EQ Curve"=w1123:T4, "Sens Curve"=w1122:T4)
                n188 = Reverse String(1:w1102) -> (0:w1106:string)
                n189 = Unbundle By Name(w1119) -> ("Calibration 2D"=w1127:T2[])
                n190 = Match Pattern(string=w1106, regular expression="[.]") -> (after substring=w1104:string)  [unwired: 4 out]
                n191 = Reverse String(1:w1104) -> (0:w1101:string)
                n192 = call "CRYGet Cal Info From SignalType and Channel Name.vi"("Calibration"=w1119, "Signal Type"=w1120, "In/Out?"=TRUE) -> ("Index"=w1121:i32)  [unwired: 6 in, 2 out]
                n193 = Index Array(array=w1127, index=w1121) -> (element=w1128:T2)
                n194 = Bundle By Name(cluster=w1128, "Corr Curve"=w1124, "EQ Curve"=w1123, "Sens Curve"=w1122, "Calibration.Calibrated Device"=w1102) -> (w1100:T2)
                n195 = Build Array(w1100) -> (w1103:T2[])
                n196 = call "CRYRepair Calibration Display.vi"("Calibration In"=w1103, "Calibration Step Name"=w1101) -> ("Calibration Out"=w1099:T2[])  [unwired: 1 in, 8 out]
                n197 = Index Array(array=w1099) -> (element=w1098:T2)  [unwired: 1 in]
                n198 = Unbundle By Name(w1098) -> ("Sens Curve.Curve"=w1108:cluster{"x":dbl, "y":dbl, "z":dbl}[], "Sens Curve.Y unit"=w1116:string, "Sens Curve.Y dB ref"=w1111:dbl, "Calibration.Sensitivity Curve Name"=w1112:string, "Calibration.Correction Curve Name"=w1113:string)
                n199 = local write "Sens Value In"(w1112) -> ()
                n200 = local write "Corre Curve In"(w1113) -> ()
                n201 = local write "Sens unit In"(w1116) -> ()
                n202 = local write "dB ref In"(w1111) -> ()
                n203 = Index Array(array=w1108, index=0) -> (element=w1110:cluster{"x":dbl, "y":dbl, "z":dbl})
                n204 = Unbundle By Name(w1110) -> ("x"=w1097:dbl, "y"=w1107:dbl)
                n205 = local write "Sensitivity In"(w1107) -> ()
                n206 = local write "Hz In"(w1097) -> ()
                n207 = Match Pattern(string=w1116, regular expression="/") -> (after substring=w1115:string)  [unwired: 4 out]
                n208 = Replace Array Subset(array=w1127, new element=w1098, index=w1121) -> (w1125:T2[])
                n209 = local write "unit In"(w1115) -> ()
                n210 = Bundle By Name(cluster=w1119, "Calibration 2D"=w1125) -> (w1126:T1)
                n211 = call "CRYConversion dB-Lin.vi"("dB ref."=1.0, "Lin In"=w1107) -> ("Log Out"=w1117:dbl)  [unwired: 4 in, 3 out]
                n212 = local write "dB In"(w1117) -> ()
                n213 = local write "Calibration"(w1126) -> ()
              }
              frame Error {
              }
            }
          }
          frame True {
            n214 = local read "Calibration"() -> (w1146:T1)
            n215 = call "CRYGet Cal Info From SignalType and Channel Name.vi"("Calibration"=w1146, "Signal Type"=w1135, "In/Out?"=TRUE) -> ("Calibration 2D Cluster"=w1161:T2, "Index"=w1145:i32)  [unwired: 6 in, 1 out]
            n216 = Unbundle By Name(w1146) -> ("Calibration 2D"=w1149:T2[])
            n217 = Unbundle By Name(w1161) -> ("Sens Curve.Curve"=w1151:cluster{"x":dbl, "y":dbl, "z":dbl}[], "Sens Curve.Y unit"=w1157:string, "Sens Curve.Y dB ref"=w1154:dbl)
            n218 = Reverse String(1:w1134) -> (0:w1144:string)
            n219 = Index Array(array=w1149, index=w1145) -> (element=w1133:T2)
            n220 = Bundle By Name(cluster=w1133, "Calibration.Calibrated Device"=w1134) -> (w1132:T2)
            n221 = Match Pattern(string=w1144, regular expression="[.]") -> (after substring=w1142:string)  [unwired: 4 out]
            n222 = local write "Sens unit In"(w1157) -> ()
            n223 = local write "dB ref In"(w1154) -> ()
            n224 = Reverse String(1:w1142) -> (0:w1139:string)
            n225 = Index Array(array=w1151, index=0) -> (element=w1153:cluster{"x":dbl, "y":dbl, "z":dbl})
            n226 = Unbundle By Name(w1153) -> ("y"=w1150:dbl)
            n227 = Build Array(w1132) -> (w1141:T2[])
            n228 = local write "Sensitivity In"(w1150) -> ()
            n229 = call "CRYRepair Calibration Display.vi"("Calibration In"=w1141, "Calibration Step Name"=w1139) -> ("Calibration Out"=w1140:T2[])  [unwired: 1 in, 8 out]
            n230 = Index Array(array=w1140) -> (element=w1136:T2)  [unwired: 1 in]
            n231 = Match Pattern(string=w1157, regular expression="/") -> (after substring=w1156:string)  [unwired: 4 out]
            n232 = Unbundle By Name(w1136) -> ("Calibration.Sensitivity Curve Name"=w1137:string, "Calibration.Correction Curve Name"=w1138:string)
            n233 = Replace Array Subset(array=w1149, new element=w1136, index=w1145) -> (w1147:T2[])
            n234 = local write "unit In"(w1156) -> ()
            n235 = call "CRYConversion dB-Lin.vi"("dB ref."=1.0, "Lin In"=w1150) -> ("Log Out"=w1158:dbl)  [unwired: 4 in, 3 out]
            n236 = Bundle By Name(cluster=w1146, "Calibration 2D"=w1147) -> (w1148:T1)
            n237 = local write "dB In"(w1158) -> ()
            n238 = local write "Calibration"(w1148) -> ()
            n239 = local write "Corre Curve In"(w1138) -> ()
            n240 = local write "Sens Value In"(w1137) -> ()
          }
        }
        n241 = property on="Units In" class="Bool"("DisabledEnum"=w1084) -> ()  [unwired: 2 in, 2 out]
        n242 = property on="I_From CurveLib" class="Bool"("DisabledEnum"=w1084) -> ()  [unwired: 2 in, 2 out]
        n243 = property on="CalibrationSeq In" class="Ring (strict)"("DisabledEnum"=w1084) -> ()  [unwired: 2 in, 2 out]
        n244 = property on="Calibrate In" class="Bool"("DisabledEnum"=w1084) -> ()  [unwired: 2 in, 2 out]
      }
      event "Calibrated Output Device": Value Change {
        n245 = event-data() -> ()  [unwired: 7 out]
        n246 = local read "Origine Calibration"() -> (w1181:T1)
        n247 = property on="Output Signal Type" class="Ring (strict)"() -> ("RingText.Text"=w1169:string)  [unwired: 2 in, 2 out]
        n248 = property on="Output Signal Type" class="Ring (strict)"() -> ("RingText.Text"=w1175:string)  [unwired: 2 in, 2 out]
        n249 = property on="Calibrated Output Device" class="Ring (strict)"() -> ("RingText.Text"=w1172:string)  [unwired: 2 in, 2 out]
        n250 = local read "Calibration"() -> (w1173:T1)
        n251 = Equal?(x=w1169, y="Mouth Sim 2") -> (x = y?=w1167:bool)
        n252 = Equal?(x=w1169, y="Mouth Sim 1") -> (x = y?=w1168:bool)
        n253 = Equal?(x=w1172, y="unity cal-out.dat") -> (x = y?=w1166:bool)
        n254 = call "CRYGet Cal Info From SignalType and Channel Name.vi"("Calibration"=w1173, "Signal Type"=w1175, "In/Out?"=FALSE) -> ("Calibration 2D Cluster"=w1179:T2)  [unwired: 6 in, 2 out]
        n255 = Unbundle By Name(w1179) -> ("Calibration.Calibrated Device"=w1180:string)
        n256 = call "CRYTest Changing State.vi"("Origine Calibration"=w1181, "New Calibration"=w1173, "Signal Type"=w1175, "In/Out?"=FALSE) -> ("Changed/Added"=w1177:bool)  [unwired: 5 in, 2 out]
        n257 = Select(t=T9."Disabled and Grayed Out" ("Disabled"), s=w1166, f=T9."Enabled" ("Disabled")) -> (s? t:f=w1163:T9)
        n258 = Compound Arithmetic op=OR(w1168, w1167) -> (w1165:bool)
        n259 = Equal?(x=w1172, y=w1180) -> (x = y?=w1174:bool)
        n260 = property on="O_Delete" class="Bool"("DisabledEnum"=w1163) -> ()  [unwired: 2 in, 2 out]
        n261 = property on="O_Rename" class="Bool"("DisabledEnum"=w1163) -> ()  [unwired: 2 in, 2 out]
        n262 = property on="Sensitivity Out" class="DigNum (strict)"("DisabledEnum"=w1163) -> ()  [unwired: 2 in, 2 out]
        n263 = And(x=w1177, y=w1174) -> (x .and. y?=w1176:bool)
        n264 = case shown="False" w1176 {
          tunnel: w1172 -> [w1186 _]
          tunnel: w1175 -> [_ w1235]
          tunnel: w1173 -> [_ w1232]
          frame False {
            n265 = global read "CRYMainGlobal.vi" "Calibration path"() -> (w1192:path)
            n266 = Concatenate Strings("Output Calibration Data" ("name or relative path"), "\\" ("string"), w1186) -> (w1188:string)
            n267 = Build Path(base path=w1192, name or relative path=w1188) -> (appended path=w1191:path)
            n268 = call "CRYFlatten Data Read.vi"("Path In"=w1191) -> ("error out"=w1187:errorcluster, "Flatten Data Out"=w1193:string)  [unwired: 6 in, 1 out]
            n269 = case shown="No Error" w1187 {
              tunnel: w1193 -> [w1231 _]
              tunnel: w1186 -> [w1216 _]
              frame No Error {
                n270 = property on="Output Signal Type" class="Ring (strict)"() -> ("RingText.Text"=w1228:string)  [unwired: 2 in, 2 out]
                n271 = local read "Calibration"() -> (w1219:T1)
                n272 = Reverse String(1:w1216) -> (0:w1215:string)
                n273 = call "CRYUnflatten Calibration Data File.vi"("Flattened Calibration"=w1231) -> ("Calibration 2D Data File Out"=w1230:T2)  [unwired: 8 in, 2 out]
                n274 = Match Pattern(string=w1215, regular expression="[.]") -> (after substring=w1218:string)  [unwired: 4 out]
                n275 = Unbundle By Name(w1230) -> ("Corr Curve"=w1220:T4, "EQ Curve"=w1221:T4, "Sens Curve"=w1222:T4)
                n276 = Unbundle By Name(w1219) -> ("Calibration 2D"=w1225:T2[])
                n277 = Reverse String(1:w1218) -> (0:w1214:string)
                n278 = call "CRYGet Cal Info From SignalType and Channel Name.vi"("Calibration"=w1219, "Signal Type"=w1228, "In/Out?"=FALSE) -> ("Index"=w1226:i32)  [unwired: 6 in, 2 out]
                n279 = Index Array(array=w1225, index=w1226) -> (element=w1227:T2)
                n280 = Bundle By Name(cluster=w1227, "Corr Curve"=w1220, "EQ Curve"=w1221, "Sens Curve"=w1222, "Calibration.Calibrated Device"=w1216) -> (w1213:T2)
                n281 = Build Array(w1213) -> (w1212:T2[])
                n282 = call "CRYRepair Calibration Display.vi"("Calibration In"=w1212, "Calibration Step Name"=w1214) -> ("Calibration Out"=w1211:T2[])  [unwired: 1 in, 8 out]
                n283 = Index Array(array=w1211) -> (element=w1199:T2)  [unwired: 1 in]
                n284 = Unbundle By Name(w1199) -> ("Sens Curve.Curve"=w1201:cluster{"x":dbl, "y":dbl, "z":dbl}[], "Sens Curve.Y unit"=w1197:string, "Sens Curve.Y dB ref"=w1204:dbl, "Calibration.Sensitivity Curve Name"=w1205:string, "Calibration.Correction Curve Name"=w1206:string, "Calibration.Equalization Curve Name"=w1210:string)
                n285 = Index Array(array=w1201, index=0) -> (element=w1203:cluster{"x":dbl, "y":dbl, "z":dbl})
                n286 = local write "Sens Value Out"(w1205) -> ()
                n287 = local write "Corre Curve Out"(w1206) -> ()
                n288 = local write "Sens unit Out"(w1197) -> ()
                n289 = local write "EQ Curve Out"(w1210) -> ()
                n290 = local write "dB ref Out"(w1204) -> ()
                n291 = Unbundle By Name(w1203) -> ("x"=w1198:dbl, "y"=w1200:dbl)
                n292 = local write "Sensitivity Out"(w1200) -> ()
                n293 = local write "Hz Out"(w1198) -> ()
                n294 = Reverse String(1:w1197) -> (0:w1196:string)
                n295 = Replace Array Subset(array=w1225, new element=w1199, index=w1226) -> (w1223:T2[])
                n296 = call "CRYConversion dB-Lin.vi"("dB ref."=1.0, "Lin In"=w1200) -> ("Log Out"=w1208:dbl)  [unwired: 4 in, 3 out]
                n297 = Match Pattern(string=w1196, regular expression="/" ("search string/char (-)")) -> (after substring=w1195:string)  [unwired: 4 out]
                n298 = Bundle By Name(cluster=w1219, "Calibration 2D"=w1223) -> (w1224:T1)
                n299 = local write "dB Out"(w1208) -> ()
                n300 = Reverse String(1:w1195) -> (0:w1194:string)
                n301 = local write "unit Out"(w1194) -> ()
                n302 = local write "Calibration"(w1224) -> ()
              }
              frame Error {
              }
            }
          }
          frame True {
            n303 = Unbundle By Name(w1232) -> ("Calibration 2D"=w1253:T2[])
            n304 = call "CRYGet Cal Info From SignalType and Channel Name.vi"("Calibration"=w1232, "Signal Type"=w1235, "In/Out?"=FALSE) -> ("Calibration 2D Cluster"=w1263:T2, "Index"=w1250:i32)  [unwired: 6 in, 1 out]
            n305 = Unbundle By Name(w1263) -> ("Sens Curve.Curve"=w1255:cluster{"x":dbl, "y":dbl, "z":dbl}[], "Sens Curve.Y unit"=w1239:string, "Sens Curve.Y dB ref"=w1258:dbl)
            n306 = Index Array(array=w1253, index=w1250) -> (element=w1233:T2)
            n307 = Unbundle By Name(w1233) -> ("Calibration.Calibrated Device"=w1234:string)
            n308 = Reverse String(1:w1234) -> (0:w1249:string)
            n309 = Match Pattern(string=w1249, regular expression="[.]") -> (after substring=w1247:string)  [unwired: 4 out]
            n310 = Reverse String(1:w1247) -> (0:w1244:string)
            n311 = Index Array(array=w1255, index=0) -> (element=w1257:cluster{"x":dbl, "y":dbl, "z":dbl})
            n312 = Build Array(w1233) -> (w1246:T2[])
            n313 = local write "Sens unit Out"(w1239) -> ()
            n314 = local write "dB ref Out"(w1258) -> ()
            n315 = Unbundle By Name(w1257) -> ("y"=w1254:dbl)
            n316 = call "CRYRepair Calibration Display.vi"("Calibration In"=w1246, "Calibration Step Name"=w1244) -> ("Calibration Out"=w1245:T2[])  [unwired: 1 in, 8 out]
            n317 = local write "Sensitivity Out"(w1254) -> ()
            n318 = Index Array(array=w1245) -> (element=w1243:T2)  [unwired: 1 in]
            n319 = Unbundle By Name(w1243) -> ("Calibration.Sensitivity Curve Name"=w1242:string, "Calibration.Correction Curve Name"=w1241:string, "Calibration.Equalization Curve Name"=w1240:string)
            n320 = Reverse String(1:w1239) -> (0:w1238:string)
            n321 = call "CRYConversion dB-Lin.vi"("dB ref."=1.0, "Lin In"=w1254) -> ("Log Out"=w1260:dbl)  [unwired: 4 in, 3 out]
            n322 = Replace Array Subset(array=w1253, new element=w1243, index=w1250) -> (w1251:T2[])
            n323 = Match Pattern(string=w1238, regular expression="/" ("search string/char (-)")) -> (after substring=w1237:string)  [unwired: 4 out]
            n324 = local write "dB Out"(w1260) -> ()
            n325 = Bundle By Name(cluster=w1232, "Calibration 2D"=w1251) -> (w1252:T1)
            n326 = Reverse String(1:w1237) -> (0:w1236:string)
            n327 = local write "unit Out"(w1236) -> ()
            n328 = local write "Calibration"(w1252) -> ()
            n329 = local write "Sens Value Out"(w1242) -> ()
            n330 = local write "Corre Curve Out"(w1241) -> ()
            n331 = local write "EQ Curve Out"(w1240) -> ()
          }
        }
        n332 = property on="Hz Out" class="DigNum (strict)"("DisabledEnum"=w1163) -> ()  [unwired: 2 in, 2 out]
        n333 = property on="dB Out" class="DigNum (strict)"("DisabledEnum"=w1163) -> ()  [unwired: 2 in, 2 out]
        n334 = property on="Units Out" class="Bool"("DisabledEnum"=w1163) -> ()  [unwired: 2 in, 2 out]
        n335 = property on="O_From CurveLib" class="Bool"("DisabledEnum"=w1163) -> ()  [unwired: 2 in, 2 out]
        n336 = Select(t=T9."Disabled and Grayed Out" ("s? t:f"), s=w1165, f=w1163) -> (s? t:f=w1162:T9)
        n337 = property on="Calibrate Out" class="Bool"("DisabledEnum"=w1163) -> ()  [unwired: 2 in, 2 out]
        n338 = property on="CalibrationSeq Out" class="Ring (strict)"("DisabledEnum"=w1162) -> ()  [unwired: 2 in, 2 out]
      }
      event "Main Tab": Value Change {
        n339 = event-data() -> ("NewVal"=w1265:enum32{"Input", "Output", "Help"})  [unwired: 6 out]
        n340 = local read "Calibration"() -> (w1266:T1)
        n341 = Bundle By Name(cluster=w1266, "Tab Value"=w1265) -> (w1264:T1)
        n342 = local write "Calibration"(w1264) -> ()
      }
      event "Channel In": Value Change {
        w1269 = "/" ("regular expression")
        n343 = event-data() -> ()  [unwired: 7 out]
        n344 = local read "Hardware In"() -> (w1293:string)
        n345 = property on="Channel In" class="Ring (strict)"() -> ("RingText.Text"=w1285:string)  [unwired: 2 in, 2 out]
        n346 = local read "Calibration"() -> (w1289:T1)
        n347 = property on="Input Signal Type" class="Ring (strict)"() -> ("RingText.Text"=w1288:string)  [unwired: 2 in, 2 out]
        n348 = call "CRYGet Channel Infor Table.vi"("Channel Name"=w1285, "Input/Output?"=TRUE, "Hardware In"=w1293) -> ("SoundCard Unit"=w1273:string, "List Item Out"=w1291:string[][])  [unwired: 6 in, 1 out]
        n349 = property on="Input Channel Info" class="MCListbox (strict)"("ItemNames"=w1291) -> ()  [unwired: 2 in, 2 out]
        n350 = Unbundle By Name(w1289) -> ("Calibration 2D"=w1287:T2[])
        n351 = call "CRYGet Cal Info From SignalType and Channel Name.vi"("Calibration"=w1289, "Signal Type"=w1288, "In/Out?"=TRUE) -> ("Index"=w1267:i32)  [unwired: 6 in, 2 out]
        n352 = Index Array(array=w1287, index=w1267) -> (element=w1286:T2)
        n353 = Bundle By Name(cluster=w1286, "Calibration.Cha Name"=w1285) -> (w1275:T2)
        n354 = Unbundle By Name(w1275) -> ("Calibration.Calibrated Device"=w1276:string, "Sens Curve.Y unit"=w1274:string)
        n355 = Reverse String(1:w1276) -> (0:w1284:string)
        n356 = Match Pattern(string=w1284, regular expression="[.]") -> (after substring=w1282:string)  [unwired: 4 out]
        n357 = Reverse String(1:w1282) -> (0:w1279:string)
        n358 = Match Pattern(string=w1274, regular expression=w1269) -> (after substring=w1268:string)  [unwired: 1 in, 3 out]
        n359 = Build Array(w1275) -> (w1281:T2[])
        n360 = call "CRYRepair Calibration Display.vi"("Calibration In"=w1281, "Calibration Step Name"=w1279) -> ("Calibration Out"=w1280:T2[])  [unwired: 1 in, 8 out]
        n361 = Index Array(array=w1280) -> (element=w1272:T2)  [unwired: 1 in]
        n362 = Concatenate Strings(w1273, w1269, w1268) -> (w1270:string)
        n363 = Bundle By Name(cluster=w1272, "Sens Curve.Y unit"=w1270) -> (w1271:T2)
        n364 = local write "Sens unit In"(w1270) -> ()
        n365 = Unbundle By Name(w1272) -> ("Calibration.Sensitivity Curve Name"=w1277:string, "Calibration.Correction Curve Name"=w1278:string)
        n366 = Replace Array Subset(array=w1287, new element=w1271, index=w1267) -> (w1294:T2[])
        n367 = Bundle By Name(cluster=w1289, "Calibration 2D"=w1294) -> (w1295:T1)
        n368 = local write "Calibration"(w1295) -> ()
        n369 = local write "Sens Value In"(w1277) -> ()
        n370 = local write "Corre Curve In"(w1278) -> ()
      }
      event "Channel Out": Value Change {
        w1298 = "/" ("regular expression")
        n371 = event-data() -> ()  [unwired: 7 out]
        n372 = local read "Hardware In"() -> (w1326:string)
        n373 = property on="Channel Out" class="Ring (strict)"() -> ("RingText.Text"=w1317:string)  [unwired: 2 in, 2 out]
        n374 = local read "Calibration"() -> (w1321:T1)
        n375 = property on="Output Signal Type" class="Ring (strict)"() -> ("RingText.Text"=w1322:string)  [unwired: 2 in, 2 out]
        n376 = call "CRYGet Channel Infor Table.vi"("Channel Name"=w1317, "Input/Output?"=FALSE, "Hardware In"=w1326) -> ("SoundCard Unit"=w1299:string, "List Item Out"=w1324:string[][])  [unwired: 6 in, 1 out]
        n377 = property on="Output Channel Info" class="MCListbox (strict)"("ItemNames"=w1324) -> ()  [unwired: 2 in, 2 out]
        n378 = Unbundle By Name(w1321) -> ("Calibration 2D"=w1320:T2[])
        n379 = call "CRYGet Cal Info From SignalType and Channel Name.vi"("Calibration"=w1321, "Signal Type"=w1322, "In/Out?"=FALSE) -> ("Index"=w1296:i32)  [unwired: 6 in, 2 out]
        n380 = Index Array(array=w1320, index=w1296) -> (element=w1318:T2)
        n381 = Bundle By Name(cluster=w1318, "Calibration.Cha Name"=w1317) -> (w1306:T2)
        n382 = Unbundle By Name(w1306) -> ("Calibration.Calibrated Device"=w1310:string, "Sens Curve.Y unit"=w1302:string)
        n383 = Reverse String(1:w1302) -> (0:w1305:string)
        n384 = Match Pattern(string=w1305, regular expression=w1298) -> (after substring=w1297:string)  [unwired: 1 in, 3 out]
        n385 = Reverse String(1:w1310) -> (0:w1316:string)
        n386 = Match Pattern(string=w1316, regular expression="[.]") -> (after substring=w1314:string)  [unwired: 4 out]
        n387 = Reverse String(1:w1297) -> (0:w1300:string)
        n388 = Reverse String(1:w1314) -> (0:w1311:string)
        n389 = Concatenate Strings(w1300, w1298, w1299) -> (w1301:string)
        n390 = Build Array(w1306) -> (w1313:T2[])
        n391 = call "CRYRepair Calibration Display.vi"("Calibration In"=w1313, "Calibration Step Name"=w1311) -> ("Calibration Out"=w1312:T2[])  [unwired: 1 in, 8 out]
        n392 = local write "Sens unit Out"(w1301) -> ()
        n393 = Index Array(array=w1312) -> (element=w1304:T2)  [unwired: 1 in]
        n394 = Bundle By Name(cluster=w1304, "Sens Curve.Y unit"=w1301) -> (w1303:T2)
        n395 = Unbundle By Name(w1304) -> ("Calibration.Sensitivity Curve Name"=w1309:string, "Calibration.Correction Curve Name"=w1308:string, "Calibration.Equalization Curve Name"=w1307:string)
        n396 = Replace Array Subset(array=w1320, new element=w1303, index=w1296) -> (w1319:T2[])
        n397 = Bundle By Name(cluster=w1321, "Calibration 2D"=w1319) -> (w1327:T1)
        n398 = local write "Sens Value Out"(w1309) -> ()
        n399 = local write "Corre Curve Out"(w1308) -> ()
        n400 = local write "EQ Curve Out"(w1307) -> ()
        n401 = local write "Calibration"(w1327) -> ()
      }
      event "Sensitivity In": Value Change {
        n402 = event-data() -> ("NewVal"=w1328:dbl)  [unwired: 6 out]
        n403 = flat-sequence {
          tunnel: w1328 -> [w1345]
          frame #0 {
            n404 = local read "Calibration"() -> (w1331:T1)
            n405 = property on="Input Signal Type" class="Ring (strict)"() -> ("RingText.Text"=w1332:string)  [unwired: 2 in, 2 out]
            n406 = Unbundle By Name(w1331) -> ("Calibration 2D"=w1335:T2[])
            n407 = call "CRYGet Cal Info From SignalType and Channel Name.vi"("Calibration"=w1331, "Signal Type"=w1332, "In/Out?"=TRUE) -> ("Index"=w1330:i32)  [unwired: 6 in, 2 out]
            n408 = Index Array(array=w1335, index=w1330) -> (element=w1340:T2)
            n409 = Unbundle By Name(w1340) -> ("Sens Curve.Curve"=w1339:cluster{"x":dbl, "y":dbl, "z":dbl}[])
            n410 = call "CRYConversion dB-Lin.vi"("dB ref."=1.0, "Lin In"=w1345) -> ("Log Out"=w1344:dbl)  [unwired: 4 in, 3 out]
            n411 = local write "Signal Type Index"(w1330) -> ()
            n412 = Index Array(array=w1339, index=0) -> (element=w1337:cluster{"x":dbl, "y":dbl, "z":dbl})
            n413 = local write "dB In"(w1344) -> ()
            n414 = Bundle By Name(cluster=w1337, "y"=w1345) -> (w1343:cluster{"x":dbl, "y":dbl, "z":dbl})
            n415 = Build Array(w1343) -> (w1342:cluster{"x":dbl, "y":dbl, "z":dbl}[])
            n416 = Bundle By Name(cluster=w1340, "Sens Curve.Curve"=w1342) -> (w1341:T2)
            n417 = Replace Array Subset(array=w1335, new element=w1341, index=w1330) -> (w1334:T2[])
            n418 = Bundle By Name(cluster=w1331, "Calibration 2D"=w1334) -> (w1329:T1)
            n419 = local write "Calibration"(w1329) -> ()
          }
          frame #1 {
            n420 = local write "Insert flag"(TRUE ("Insert flag")) -> ()
          }
        }
      }
      event "Sensitivity Out": Value Change {
        n421 = event-data() -> ("NewVal"=w1347:dbl)  [unwired: 6 out]
        n422 = flat-sequence {
          tunnel: w1347 -> [w1364]
          frame #0 {
            n423 = local read "Calibration"() -> (w1349:T1)
            n424 = property on="Output Signal Type" class="Ring (strict)"() -> ("RingText.Text"=w1350:string)  [unwired: 2 in, 2 out]
            n425 = Unbundle By Name(w1349) -> ("Calibration 2D"=w1354:T2[])
            n426 = call "CRYGet Cal Info From SignalType and Channel Name.vi"("Calibration"=w1349, "Signal Type"=w1350, "In/Out?"=FALSE) -> ("Index"=w1348:i32)  [unwired: 6 in, 2 out]
            n427 = call "CRYConversion dB-Lin.vi"("dB ref."=1.0, "Lin In"=w1364) -> ("Log Out"=w1363:dbl)  [unwired: 4 in, 3 out]
            n428 = Index Array(array=w1354, index=w1348) -> (element=w1359:T2)
            n429 = local write "dB Out"(w1363) -> ()
            n430 = Unbundle By Name(w1359) -> ("Sens Curve.Curve"=w1358:cluster{"x":dbl, "y":dbl, "z":dbl}[])
            n431 = local write "Signal Type Index"(w1348) -> ()
            n432 = Index Array(array=w1358, index=0) -> (element=w1356:cluster{"x":dbl, "y":dbl, "z":dbl})
            n433 = Bundle By Name(cluster=w1356, "y"=w1364) -> (w1362:cluster{"x":dbl, "y":dbl, "z":dbl})
            n434 = Build Array(w1362) -> (w1361:cluster{"x":dbl, "y":dbl, "z":dbl}[])
            n435 = Bundle By Name(cluster=w1359, "Sens Curve.Curve"=w1361) -> (w1360:T2)
            n436 = Replace Array Subset(array=w1354, new element=w1360, index=w1348) -> (w1353:T2[])
            n437 = Bundle By Name(cluster=w1349, "Calibration 2D"=w1353) -> (w1352:T1)
            n438 = local write "Calibration"(w1352) -> ()
          }
          frame #1 {
            n439 = local write "Insert flag"(TRUE ("Insert flag")) -> ()
          }
        }
      }
      event "Hz In": Value Change {
        n440 = event-data() -> ("NewVal"=w1366:dbl)  [unwired: 6 out]
        n441 = flat-sequence {
          tunnel: w1366 -> [w1381]
          frame #0 {
            n442 = property on="Input Signal Type" class="Ring (strict)"() -> ("RingText.Text"=w1369:string)  [unwired: 2 in, 2 out]
            n443 = local read "Calibration"() -> (w1368:T1)
            n444 = Unbundle By Name(w1368) -> ("Calibration 2D"=w1373:T2[])
            n445 = call "CRYGet Cal Info From SignalType and Channel Name.vi"("Calibration"=w1368, "Signal Type"=w1369, "In/Out?"=TRUE) -> ("Index"=w1367:i32)  [unwired: 6 in, 2 out]
            "Signal Type Index" <- w1367
            n446 = Index Array(array=w1373, index=w1367) -> (element=w1377:T2)
            n447 = Unbundle By Name(w1377) -> ("Sens Curve.Curve"=w1376:cluster{"x":dbl, "y":dbl, "z":dbl}[])
            n448 = Index Array(array=w1376, index=0) -> (element=w1374:cluster{"x":dbl, "y":dbl, "z":dbl})
            n449 = Bundle By Name(cluster=w1374, "x"=w1381) -> (w1380:cluster{"x":dbl, "y":dbl, "z":dbl})
            n450 = Build Array(w1380) -> (w1379:cluster{"x":dbl, "y":dbl, "z":dbl}[])
            n451 = Bundle By Name(cluster=w1377, "Sens Curve.Curve"=w1379) -> (w1378:T2)
            n452 = Replace Array Subset(array=w1373, new element=w1378, index=w1367) -> (w1372:T2[])
            n453 = Bundle By Name(cluster=w1368, "Calibration 2D"=w1372) -> (w1371:T1)
            n454 = local write "Calibration"(w1371) -> ()
          }
          frame #1 {
            n455 = local write "Insert flag"(TRUE ("Insert flag")) -> ()
          }
        }
      }
      event "Hz Out": Value Change {
        n456 = event-data() -> ("NewVal"=w1383:dbl)  [unwired: 6 out]
        n457 = flat-sequence {
          tunnel: w1383 -> [w1398]
          frame #0 {
            n458 = local read "Calibration"() -> (w1385:T1)
            n459 = property on="Input Signal Type" class="Ring (strict)"() -> ("RingText.Text"=w1386:string)  [unwired: 2 in, 2 out]
            n460 = Unbundle By Name(w1385) -> ("Calibration 2D"=w1390:T2[])
            n461 = call "CRYGet Cal Info From SignalType and Channel Name.vi"("Calibration"=w1385, "Signal Type"=w1386, "In/Out?"=FALSE) -> ("Index"=w1384:i32)  [unwired: 6 in, 2 out]
            n462 = Index Array(array=w1390, index=w1384) -> (element=w1394:T2)
            n463 = Unbundle By Name(w1394) -> ("Sens Curve.Curve"=w1393:cluster{"x":dbl, "y":dbl, "z":dbl}[])
            n464 = local write "Signal Type Index"(w1384) -> ()
            n465 = Index Array(array=w1393, index=0) -> (element=w1391:cluster{"x":dbl, "y":dbl, "z":dbl})
            n466 = Bundle By Name(cluster=w1391, "x"=w1398) -> (w1397:cluster{"x":dbl, "y":dbl, "z":dbl})
            n467 = Build Array(w1397) -> (w1396:cluster{"x":dbl, "y":dbl, "z":dbl}[])
            n468 = Bundle By Name(cluster=w1394, "Sens Curve.Curve"=w1396) -> (w1395:T2)
            n469 = Replace Array Subset(array=w1390, new element=w1395, index=w1384) -> (w1389:T2[])
            n470 = Bundle By Name(cluster=w1385, "Calibration 2D"=w1389) -> (w1388:T1)
            n471 = local write "Calibration"(w1388) -> ()
          }
          frame #1 {
            n472 = local write "Insert flag"(TRUE ("Insert flag")) -> ()
          }
        }
      }
      event "dB In": Value Change {
        n473 = event-data() -> ("NewVal"=w1400:dbl)  [unwired: 6 out]
        n474 = flat-sequence {
          tunnel: w1400 -> [w1417]
          frame #0 {
            n475 = local read "Calibration"() -> (w1402:T1)
            n476 = property on="Input Signal Type" class="Ring (strict)"() -> ("RingText.Text"=w1403:string)  [unwired: 2 in, 2 out]
            n477 = Unbundle By Name(w1402) -> ("Calibration 2D"=w1407:T2[])
            n478 = call "CRYGet Cal Info From SignalType and Channel Name.vi"("Calibration"=w1402, "Signal Type"=w1403, "In/Out?"=TRUE) -> ("Index"=w1401:i32)  [unwired: 6 in, 2 out]
            n479 = local write "Signal Type Index"(w1401) -> ()
            n480 = Index Array(array=w1407, index=w1401) -> (element=w1412:T2)
            n481 = Unbundle By Name(w1412) -> ("Sens Curve.Curve"=w1411:cluster{"x":dbl, "y":dbl, "z":dbl}[])
            n482 = call "CRYConversion dB-Lin.vi"("dB ref."=1.0, "Log In"=w1417) -> ("Lin Out"=w1413:dbl)  [unwired: 4 in, 3 out]
            n483 = Index Array(array=w1411, index=0) -> (element=w1409:cluster{"x":dbl, "y":dbl, "z":dbl})
            n484 = Bundle By Name(cluster=w1409, "y"=w1413) -> (w1415:cluster{"x":dbl, "y":dbl, "z":dbl})
            n485 = local write "Sensitivity In"(w1413) -> ()
            n486 = Build Array(w1415) -> (w1414:cluster{"x":dbl, "y":dbl, "z":dbl}[])
            n487 = Bundle By Name(cluster=w1412, "Sens Curve.Curve"=w1414) -> (w1416:T2)
            n488 = Replace Array Subset(array=w1407, new element=w1416, index=w1401) -> (w1406:T2[])
            n489 = Bundle By Name(cluster=w1402, "Calibration 2D"=w1406) -> (w1405:T1)
            n490 = local write "Calibration"(w1405) -> ()
          }
          frame #1 {
            n491 = local write "Insert flag"(TRUE ("Insert flag")) -> ()
          }
        }
      }
      event "dB Out": Value Change {
        n492 = event-data() -> ("NewVal"=w1419:dbl)  [unwired: 6 out]
        n493 = flat-sequence {
          tunnel: w1419 -> [w1436]
          frame #0 {
            n494 = local read "Calibration"() -> (w1421:T1)
            n495 = property on="Output Signal Type" class="Ring (strict)"() -> ("RingText.Text"=w1422:string)  [unwired: 2 in, 2 out]
            n496 = Unbundle By Name(w1421) -> ("Calibration 2D"=w1426:T2[])
            n497 = call "CRYGet Cal Info From SignalType and Channel Name.vi"("Calibration"=w1421, "Signal Type"=w1422, "In/Out?"=FALSE) -> ("Index"=w1420:i32)  [unwired: 6 in, 2 out]
            n498 = local write "Signal Type Index"(w1420) -> ()
            n499 = Index Array(array=w1426, index=w1420) -> (element=w1431:T2)
            n500 = Unbundle By Name(w1431) -> ("Sens Curve.Curve"=w1430:cluster{"x":dbl, "y":dbl, "z":dbl}[])
            n501 = call "CRYConversion dB-Lin.vi"("dB ref."=1.0, "Log In"=w1436) -> ("Lin Out"=w1432:dbl)  [unwired: 4 in, 3 out]
            n502 = local write "Sensitivity Out"(w1432) -> ()
            n503 = Index Array(array=w1430, index=0) -> (element=w1428:cluster{"x":dbl, "y":dbl, "z":dbl})
            n504 = Bundle By Name(cluster=w1428, "y"=w1432) -> (w1435:cluster{"x":dbl, "y":dbl, "z":dbl})
            n505 = Build Array(w1435) -> (w1434:cluster{"x":dbl, "y":dbl, "z":dbl}[])
            n506 = Bundle By Name(cluster=w1431, "Sens Curve.Curve"=w1434) -> (w1433:T2)
            n507 = Replace Array Subset(array=w1426, new element=w1433, index=w1420) -> (w1425:T2[])
            n508 = Bundle By Name(cluster=w1421, "Calibration 2D"=w1425) -> (w1424:T1)
            n509 = local write "Calibration"(w1424) -> ()
          }
          frame #1 {
            n510 = local write "Insert flag"(TRUE ("Insert flag")) -> ()
          }
        }
      }
      event "Help": Value Change {
        n511 = event-data() -> ("NewVal"=w1439:string)  [unwired: 6 out]
        n512 = local read "Calibration"() -> (w1440:T1)
        n513 = Bundle By Name(cluster=w1440, "Help"=w1439) -> (w1438:T1)
        n514 = local write "Calibration"(w1438) -> ()
      }
      event "CalibrationSeq In": Value Change {
        n515 = event-data() -> ("NewVal"=w1441:u16)  [unwired: 6 out]
        n516 = flat-sequence {
          tunnel: w1441 -> [w1452]
          frame #0 {
            n517 = local read "Calibration"() -> (w1443:T1)
            n518 = property on="Input Signal Type" class="Ring (strict)"() -> ("RingText.Text"=w1444:string)  [unwired: 2 in, 2 out]
            n519 = property on="CalibrationSeq In" class="Ring (strict)"() -> ("Strings []"=w1453:string[])  [unwired: 2 in, 2 out]
            n520 = Unbundle By Name(w1443) -> ("Calibration 2D"=w1448:T2[])
            n521 = call "CRYGet Cal Info From SignalType and Channel Name.vi"("Calibration"=w1443, "Signal Type"=w1444, "In/Out?"=TRUE) -> ("Index"=w1442:i32)  [unwired: 6 in, 2 out]
            n522 = Index Array(array=w1453, index=w1452) -> (element=w1450:string)
            n523 = local write "Signal Type Index"(w1442) -> ()
            n524 = Index Array(array=w1448, index=w1442) -> (element=w1451:T2)
            n525 = Bundle By Name(cluster=w1451, "Calibration.Device"=w1450) -> (w1449:T2)
            n526 = Replace Array Subset(array=w1448, new element=w1449, index=w1442) -> (w1447:T2[])
            n527 = Bundle By Name(cluster=w1443, "Calibration 2D"=w1447) -> (w1446:T1)
            n528 = local write "Calibration"(w1446) -> ()
          }
          frame #1 {
            n529 = local write "Insert flag"(TRUE ("Insert flag")) -> ()
          }
        }
      }
      event "CalibrationSeq Out": Value Change {
        n530 = event-data() -> ("NewVal"=w1455:u16)  [unwired: 6 out]
        n531 = flat-sequence {
          tunnel: w1455 -> [w1464]
          frame #0 {
            n532 = property on="Output Signal Type" class="Ring (strict)"() -> ("RingText.Text"=w1458:string)  [unwired: 2 in, 2 out]
            n533 = local read "Calibration"() -> (w1457:T1)
            n534 = call "CRYGet Cal Info From SignalType and Channel Name.vi"("Calibration"=w1457, "Signal Type"=w1458, "In/Out?"=FALSE) -> ("Index"=w1456:i32)  [unwired: 6 in, 2 out]
            n535 = property on="CalibrationSeq Out" class="Ring (strict)"() -> ("Strings []"=w1465:string[])  [unwired: 2 in, 2 out]
            n536 = Unbundle By Name(w1457) -> ("Calibration 2D"=w1462:T2[])
            n537 = Index Array(array=w1465, index=w1464) -> (element=w1463:string)
            n538 = Index Array(array=w1462, index=w1456) -> (element=w1467:T2)
            n539 = local write "Signal Type Index"(w1456) -> ()
            n540 = Bundle By Name(cluster=w1467, "Calibration.Device"=w1463) -> (w1466:T2)
            n541 = Replace Array Subset(array=w1462, new element=w1466, index=w1456) -> (w1461:T2[])
            n542 = Bundle By Name(cluster=w1457, "Calibration 2D"=w1461) -> (w1460:T1)
            n543 = local write "Calibration"(w1460) -> ()
          }
          frame #1 {
            n544 = local write "Insert flag"(TRUE ("Insert flag")) -> ()
          }
        }
      }
      event Pane Size {
        n545 = event-data() -> ()  [unwired: 7 out]
        n546 = control-ref of="Board Tab"() -> (w1470:refnum<vi>)
        n547 = control-ref of="This VI"() -> (w1469:refnum<vi>)
        n548 = call "CRYAlign Steps VI Center.vi"("Tab2"=w1470, "Input/Output"=TRUE ("Preview"), "VIRef"=w1469) -> ()  [unwired: 1 in, 8 out]
      }
    }
    n549 = global read "CRYMain Sub Window Global.vi" "gStop"() -> (w63:bool)
    n550 = Or(x=w63, y="stop") -> (x .or. y?=w62:bool)
    n551 = Bundle("Load Test"="Load Test", "Units In"="Units In", "Calibrate In"="Calibrate In", "Units Out"="Units Out", "Calibrate Out"="Calibrate Out", "Open_table"="Open_table", "Insert flag"="Insert flag", "Cal_ValueChange"="Cal_ValueChange", "I_Add"="I_Add", "I_Delete"="I_Delete", "I_Rename"="I_Rename", "I_Copy"="I_Copy", "O_Add"="O_Add", "O_Delete"="O_Delete", "O_Rename"="O_Rename", "O_Copy"="O_Copy", "I_SAdd"="I_SAdd", "I_SDelete"="I_SDelete", "I_SRename"="I_SRename", "I_SCopy"="I_SCopy", "O_SAdd"="O_SAdd", "O_SDelete"="O_SDelete", "O_SRename"="O_SRename", "O_SCopy"="O_SCopy", "I_From CurveLib"="I_From CurveLib", "O_From CurveLib"="O_From CurveLib", "SaveCalibration"="SaveCalibration", "Cancel"="Cancel") -> (w68:T10)  [unwired: 1 out]
    n552 = Cluster To Array(cluster=w68) -> (array=w69:bool[])
    n553 = Search 1D Array(1D array=w69, element=TRUE) -> (index of element=w59:i32)  [unwired: 1 out]
    n554 = case shown="4" w59 {
      selector: w59 -> [_ _ _ _ _ _ _ _ w520 w735 w887 _ _ _]
      tunnel: "Open_table" -> [_ _ _ _ _ w470 _ _ _ _ _ _ _ _]
      tunnel: w40 -> [w82 _ _ _ _ _ _ _ _ _ _ _ _ _]
      frame 0 {
        n555 = flat-sequence {
          tunnel: w82 -> [w89]
          tunnel: [w88] -> w81
          tunnel: [w87] -> w79
          tunnel: [w83] -> w77
          tunnel: [w83] -> w75
          tunnel: w81 -> [w99]
          tunnel: [w99] -> w80
          tunnel: w79 -> [w98]
          tunnel: [w98] -> w78
          tunnel: w77 -> [w97]
          tunnel: [w97] -> w76
          tunnel: w75 -> [w94]
          tunnel: w80 -> [w128]
          tunnel: w78 -> [w127]
          tunnel: w76 -> [w124]
          frame #0 {
            n556 = local read "Calibration"() -> (w84:T1)
            n557 = call "CRYUnflatten SoundCard.vi"("Flatten SoundCard"=w89) -> ("SoundCard"=w91:T11)  [unwired: 8 in, 2 out]
            n558 = Unbundle By Name(w84) -> ("Input Signal Type"=w88:string, "Output Signal Type"=w87:string, "Help"=w92:string, "Tab Value"=w93:i32, "Calibration 2D"=w86:T2[])
            n559 = Unbundle By Name(w91) -> ("Channel Array"=w90:T12[])
            n560 = local write "Help"(w92) -> ()
            n561 = property on="Main Tab" class="TabCtl (strict)"("Value"=w93) -> ()  [unwired: 2 in, 2 out]
            n562 = call "CRYGet Diff Channel Name.vi"("Hardware Channel Array"=w90, "Calibration 2D Array In"=w86) -> ("Corrected Calibration 2D Array Out"=w85:T2[])  [unwired: 9 in]
            n563 = Bundle By Name(cluster=w84, "Calibration 2D"=w85) -> (w83:T1)
            n564 = local write "Origine Calibration"(w83) -> ()
            n565 = local write "Calibration"(w83) -> ()
          }
          frame #1 {
            n566 = call "CRYGet IO Signal Type Name.vi"("Calibration"=w94) -> ("Output Signal Type  Name Out"=w95:string[], "Input Signal Type Name Out"=w96:string[])  [unwired: 9 in]
            n567 = property on="Output Signal Type" class="Ring (strict)"("Strings []"=w95) -> ()  [unwired: 2 in, 2 out]
            n568 = property on="Input Signal Type" class="Ring (strict)"("Strings []"=w96) -> ()  [unwired: 2 in, 2 out]
          }
          frame #2 {
            w100 = enum16{"Load", "SaveAs", "Revert"}."Load" ("Mode")
            w121 = enum16{"Load", "SaveAs", "Revert"}."Load" ("Mode")
            n569 = property on="O_Signal Type Name" class="Arr (strict)"() -> ("Value"=w122:string[][])  [unwired: 2 in, 2 out]
            n570 = property on="I_Signal Type Name" class="Arr (strict)"() -> ("Value"=w123:string[][])  [unwired: 2 in, 2 out]
            n571 = property on="O_Calibrated Device Name" class="Arr (strict)"() -> ("Value"=w117:string[][])  [unwired: 2 in, 2 out]
            n572 = property on="I_Calibrated Device Name" class="Arr (strict)"() -> ("Value"=w118:string[][])  [unwired: 2 in, 2 out]
            n573 = call "CRYGet IO Signal Type Name.vi"("Calibration"=w124) -> ("Output Signal Type  Name Out"=w129:string[], "Input Signal Type Name Out"=w130:string[])  [unwired: 9 in]
            n574 = call "CRYGet Calibrated Device Name.vi"("Calibration"=w124) -> ("I_Signal Type Out"=w112:string[], "O_Signal Type Out"=w105:string[], "I_Name Out(Input Calibrated Name Out)"=w113:string[][], "O_Name Out(Output Calibrated Name Out)"=w116:string[][])  [unwired: 7 in, 4 out]
            n575 = Array Size(array=w112) -> (size(s)=w111:i32)
            n576 = Search 1D Array(1D array=w130, element=w128) -> (index of element=w126:i32)  [unwired: 1 in]
            n577 = Search 1D Array(1D array=w129, element=w127) -> (index of element=w125:i32)  [unwired: 1 in]
            n578 = Array Size(array=w105) -> (size(s)=w106:i32)
            n579 = Initialize Array("O", w111) -> (w109:string[])
            n580 = property on="Input Signal Type" class="Ring (strict)"("Val(Sgnl)"=w126) -> ()  [unwired: 2 in, 2 out]
            n581 = property on="Output Signal Type" class="Ring (strict)"("Val(Sgnl)"=w125) -> ()  [unwired: 2 in, 2 out]
            n582 = Initialize Array("O", w106) -> (w108:string[])
            n583 = Build Array(w112, w112, w109) -> (w104:string[][])
            n584 = Build Array(w105, w105, w108) -> (w102:string[][])
            n585 = Transpose 2D Array(2D array=w104) -> (transposed array=w103:string[][])
            n586 = call "CRYSet Channel State.vi"("New Name In"=w113, "Old Name In"=w118, "Mode"=w100) -> ("Name Out"=→"I_Calibrated Device Name":string[][])  [unwired: 8 in]
            n587 = call "CRYSet Channel State.vi"("New Name In"=w116, "Old Name In"=w117, "Mode"=w100) -> ("Name Out"=→"O_Calibrated Device Name":string[][])  [unwired: 8 in]
            n588 = Transpose 2D Array(2D array=w102) -> (transposed array=w101:string[][])
            n589 = call "CRYSet Channel State.vi"("New Name In"=w103, "Old Name In"=w123, "Mode"=w121) -> ("Name Out"=→"I_Signal Type Name":string[][])  [unwired: 8 in]
            n590 = call "CRYSet Channel State.vi"("New Name In"=w101, "Old Name In"=w122, "Mode"=w121) -> ("Name Out"=→"O_Signal Type Name":string[][])  [unwired: 8 in]
          }
          frame #3 {
            n591 = local read "AddStep"() -> (w131:bool)
            n592 = control-ref of="Board Tab"() -> (w133:refnum<vi>)
            n593 = control-ref of="This VI"() -> (w132:refnum<vi>)
            n594 = case shown="True" w131 {
              frame False {
              }
              frame True {
                n595 = local write "Mode"("AddStep" ("Mode")) -> ()
              }
            }
            n596 = call "CRYAlign Steps VI Center.vi"("Tab2"=w133, "Input/Output"=TRUE ("Preview"), "VIRef"=w132) -> ()  [unwired: 1 in, 8 out]
          }
          frame #4 {
            n597 = local write "AddStep"(FALSE ("AddStep")) -> ()
            n598 = local write "Load Test"(FALSE ("Load Test")) -> ()
            n599 = property on="Board Tab" class="TabCtl (strict)"("Visible"=TRUE) -> ()  [unwired: 2 in, 2 out]
            n600 = local read "Mode"() -> (w137:string)
            n601 = case shown="\"AddStep\", \"Load\", \"Revert\"" w137 {
              frame "", Default {
              }
              frame "AddStep", "Load", "Revert" {
                n602 = property on="I_Signal Type Name" class="Arr (strict)"() -> ("Value"=w148:string[][])  [unwired: 2 in, 2 out]
                n603 = property on="I_Calibrated Device Name" class="Arr (strict)"() -> ("Value"=w142:string[][])  [unwired: 2 in, 2 out]
                n604 = property on="O_Calibrated Device Name" class="Arr (strict)"() -> ("Value"=w141:string[][])  [unwired: 2 in, 2 out]
                n605 = property on="O_Signal Type Name" class="Arr (strict)"() -> ("Value"=w147:string[][])  [unwired: 2 in, 2 out]
                n606 = local read "Proper VI No"() -> (w150:i32)
                n607 = local read "Hardware In"() -> (w140:string)
                n608 = local read "Calibration"() -> (w151:T1)
                n609 = call "CRYCalibration.vi"("O_Signal Type Old In"=w147, "I_Signal Type Old In"=w148, "Hardware In"=w140, "O_Calibrated Device Name Old In"=w141, "I_Calibrated Device Name Old In"=w142, "Calibration"=w151, "Proper VI No In"=w150) -> ("O_Calibrated Device Name Out"=w143:string[][], "I_Calibrated Device Name Out"=w144:string[][], "O_Signal Type Out"=w145:string[][], "I_Signal Type Out"=w146:string[][])  [unwired: 1 in]
                n610 = property on="I_Signal Type Name" class="Arr (strict)"("Value"=w146) -> ()  [unwired: 2 in, 2 out]
                n611 = property on="I_Calibrated Device Name" class="Arr (strict)"("Value"=w144) -> ()  [unwired: 2 in, 2 out]
                n612 = property on="O_Calibrated Device Name" class="Arr (strict)"("Value"=w143) -> ()  [unwired: 2 in, 2 out]
                n613 = property on="O_Signal Type Name" class="Arr (strict)"("Value"=w145) -> ()  [unwired: 2 in, 2 out]
                n614 = local write "Mode"("" ("Mode")) -> ()
              }
            }
          }
        }
      }
      frame 1 {
        n615 = local read "dB ref In"() -> (w157:dbl)
        n616 = local read "unit In"() -> (w158:string)
        n617 = call "CRYUnits setup.vi"("Scale visible?"=FALSE, "dB/Lin"=u16 0 ("Scale"), "Unit:"=w158, "dB ref:"=w157, "Custom unit settings"=T7 {"Custom units dialog?"=FALSE, "Use custom unit?"=FALSE}, "Common dB ref."=u16 0) -> ("New unit Lin"=w160:string, "New dB ref"=w159:dbl, "Cancelled?"=w153:bool)  [unwired: 2 in, 5 out]
        n618 = case shown="False" w153 {
          tunnel: w160 -> [w162 _]
          tunnel: w159 -> [w161 _]
          frame False {
            n619 = flat-sequence {
              tunnel: w162 -> [w181]
              tunnel: w161 -> [w180]
              frame #0 {
                n620 = local write "dB ref In"(w180) -> ()
                n621 = local write "unit In"(w181) -> ()
                n622 = property on="Input Signal Type" class="Ring (strict)"() -> ("RingText.Text"=w163:string)  [unwired: 2 in, 2 out]
                n623 = local read "Calibration"() -> (w165:T1)
                n624 = call "CRYGet IOCalibration 2D.vi"("Calibration"=w165) -> ("O_Calibration 2D Out"=w168:T2[], "I_Calibration 2D Out"=w169:T2[])  [unwired: 9 in]
                n625 = call "CRYGet Calibration 2D From Signal Type.vi"("I/O Calibration 2D"=w169, "Signal Type Name In"=w163) -> ("equal Index Out"=w171:i32)  [unwired: 8 in, 1 out]
                n626 = call "CRYGet Cal Info From SignalType and Channel Name.vi"("Calibration"=w165, "Signal Type"=w163, "In/Out?"=TRUE) -> ("Index"=w164:i32)  [unwired: 6 in, 2 out]
                n627 = Index Array(array=w169, index=w171) -> (element=w178:T2)
                n628 = local write "Signal Type Index"(w164) -> ()
                n629 = Unbundle By Name(w178) -> ("Sens Curve.Y unit"=w177:string)
                n630 = Match Pattern(string=w177, regular expression="/") -> (before substring=w175:string, match substring=w174:string)  [unwired: 1 in, 2 out]
                n631 = Concatenate Strings(w175, w174, w181) -> (w173:string)
                n632 = Bundle By Name(cluster=w178, "Sens Curve.Y dB ref"=w180, "Sens Curve.Y unit"=w173) -> (w179:T2)
                n633 = local write "Sens unit In"(w173) -> ()
                n634 = Replace Array Subset(array=w169, new element=w179, index=w171) -> (w167:T2[])
                n635 = Build Array (concatenate)(w168, w167) -> (w170:T2[])
                n636 = Bundle By Name(cluster=w165, "Calibration 2D"=w170) -> (w172:T1)
                n637 = local write "Calibration"(w172) -> ()
              }
              frame #1 {
                n638 = local write "Insert flag"(TRUE ("Insert flag")) -> ()
              }
            }
          }
          frame True {
          }
        }
      }
      frame 2 {
        n639 = flat-sequence {
          tunnel: [w193] -> w186
          tunnel: [w190] -> w185
          tunnel: [w189] -> w183
          tunnel: w186 -> [w271]
          tunnel: w185 -> [w269]
          tunnel: [w269] -> w184
          tunnel: w183 -> [w270]
          tunnel: w184 -> [w293]
          frame #0 {
            n640 = property on="CalibrationSeq In" class="Ring (strict)"() -> ("Value"=w188:u16)  [unwired: 2 in, 2 out]
            n641 = stacked-sequence {
              tunnel: [w230 _ _ _] -> w192
              tunnel: [_ w239 _ _] -> w191
              tunnel: w188 -> [_ _ _ _]
              frame #0 {
                # "????????"
                n642 = local read "Calibration"() -> (w231:T1)
                n643 = call "CRYFlatten Calibration 2D.vi"("Calibration All Cluster"=w231) -> ("Calibration flattened"=w230:string)  [unwired: 10 out]
                n644 = disable-structure shown="Disabled" {
                  disable-tunnel: w230 -> [w232 _]
                  frame Disabled {
                    n645 = local read "Proper VI No"() -> (w235:i32)
                    n646 = call "CRYPreUpdate Sequence.vi"("EventName"="SequenceUpdate", "Proper VI No"=w235, "Project View Step Name Identifier Arg1"="", "Step flattened Arg2"=w232, "AllChangeFlg"=TRUE ("Name/Identifier")) -> ()  [unwired: 11 in]
                  }
                  frame Enabled {
                  }
                }
              }
              frame #1 {
                w238 = TRUE ("Calibrate")
                # "????????"
                n647 = global read "CRYMisc vis settings global.vi" "Signal Gen'r settings"() -> (w246:T13)
                n648 = Bundle By Name(cluster=w246, "gen'r mode"=0, "Play Sine Wave"=0, "frequency"=u32 1000, "output level"=0.03) -> (w241:T13)
                n649 = global write "CRYCal Global.vi" "Calibrate"(TRUE ("Calibrate")) -> ()
                n650 = global write "CRYMisc vis settings global.vi" "Menu?"(FALSE ("Menu?")) -> ()
                n651 = global write "CRYMisc vis settings global.vi" "Signal Gen'r settings"(w241) -> ()
                n652 = Bundle("Calibrate"=FALSE, "Calibrate"=w238, "Calibrate"=w238) -> (w239:T14)  [unwired: 1 out]
              }
              frame #2 {
                n653 = global read "CRYMisc vis settings global.vi" "Voltmeter Settings"() -> (w251:T15)
                n654 = Bundle By Name(cluster=w251, "rec time (sec)"=0.5, "lin/exp avg"=u16 0) -> (w250:T15)
                n655 = global write "CRYMisc vis settings global.vi" "Voltmeter Settings"(w250) -> ()
                n656 = global write "CRYCal Global.vi" "Sens In"(1.0 ("Sens In")) -> ()
              }
              frame #3 {
                n657 = local read "Hardware In"() -> (w259:string)
                n658 = local read "Calibration"() -> (w261:T1)
                n659 = property on="Input Signal Type" class="Ring (strict)"() -> ("RingText.Text"=w262:string)  [unwired: 2 in, 2 out]
                n660 = property on="Output Signal Type" class="Ring (strict)"() -> ("RingText.Text"=w265:string)  [unwired: 2 in, 2 out]
                n661 = property on="Channel Out" class="Ring (strict)"() -> ("Value"=w256:i32)  [unwired: 2 in, 2 out]
                n662 = property on="Channel In" class="Ring (strict)"() -> ("Value"=w255:i32)  [unwired: 2 in, 2 out]
                n663 = property on="Output Signal Type" class="Ring (strict)"() -> ("Value"=w267:i32)  [unwired: 2 in, 2 out]
                n664 = property on="Input Signal Type" class="Ring (strict)"() -> ("Value"=w268:i32)  [unwired: 2 in, 2 out]
                n665 = global write "CRYCal Global.vi" "Signal Type In"(w268) -> ()
                n666 = global write "CRYCal Global.vi" "Signal Type Out"(w267) -> ()
                n667 = call "CRYGet Hardware IO Infor.vi"("Hardware setup In"=w259) -> ("I_channel Info Out"=w257:T12[], "O_channel Info Out"=w258:T12[])  [unwired: 9 out]
                n668 = Index Array(array=w258, index=w256) -> (element=w254:T12)
                n669 = Index Array(array=w257, index=w255) -> (element=w253:T12)
                n670 = global write "CRYCal Global.vi" "Output Hardware Cal"(w254) -> ()
                n671 = call "CRYGet Cal Info From SignalType and Channel Name.vi"("Calibration"=w261, "Signal Type"=w262, "In/Out?"=TRUE) -> ("Calibration 2D Cluster"=w260:T2)  [unwired: 6 in, 2 out]
                n672 = call "CRYGet Cal Info From SignalType and Channel Name.vi"("Calibration"=w261, "Signal Type"=w265, "In/Out?"=FALSE) -> ("Calibration 2D Cluster"=w264:T2)  [unwired: 6 in, 2 out]
                n673 = global write "CRYCal Global.vi" "Input Hardware Cal"(w253) -> ()
                n674 = global write "CRYCal Global.vi" "Output Cal"(w264) -> ()
                n675 = global write "CRYCal Global.vi" "Input Cal"(w260) -> ()
              }
            }
            n676 = local read "Sensitivity In"() -> (w194:dbl)
            n677 = local read "Hardware In"() -> (w195:string)
            n678 = case shown="2" u16 2 ("Signal Type In") {
              tunnel: w195 -> [w203 w209 w226]
              tunnel: w194 -> [w199 w213 w222]
              tunnel: [w197 w212 w225] -> w193
              tunnel: w192 -> [w204 w211 _]
              tunnel: w191 -> [_ w210 _]
              tunnel: [w200 w206 w223] -> w190
              tunnel: [w196 w205 w220] -> w189
              frame 0, Default {
                # "Direct Cal"
                n679 = call "CRYMultimeter.vi"("Calibration in"=w204, "Hardware in"=w203, "Manual"=FALSE) -> ("Canceled?"=w200:bool, "InputLevel Out"=w201:T16)  [unwired: 8 in, 7 out]
                n680 = Unbundle By Name(w201) -> ("InputLevel"=w198:dbl)
                n681 = Select(t=w199, s=w200, f=w198) -> (s? t:f=w197:dbl)
                n682 = local read "Hz In"() -> (w196:dbl)
              }
              frame 1 {
                w215 = FALSE ("Manual")
                # "Attenuator Cal"
                n683 = call "CRYSignal Generator.vi"("Manual"=w215, "Execution control"=w210, "Hardware in"=w209, "Calibration in"=w211) -> ("Freq Out"=w205:dbl, "Amp Out"=w214:dbl)  [unwired: 6 in, 4 out]
                n684 = call "CRYMultimeter.vi"("Calibration in"=w211, "Hardware in"=w209, "Manual"=w215) -> ("Canceled?"=w206:bool, "InputLevel Out"=w208:T16)  [unwired: 8 in, 7 out]
                n685 = Unbundle By Name(w208) -> ("InputLevel"=w207:dbl)
                n686 = case shown="False" w206 {
                  tunnel: w214 -> [w217 _]
                  tunnel: w213 -> [_ w219]
                  tunnel: w207 -> [w216 _]
                  tunnel: [w218 w219] -> w212
                  frame False {
                    n687 = Divide(x=w216, y=w217) -> (x/y=w218:dbl)
                  }
                  frame True {
                  }
                }
              }
              frame 2 {
                # "Microphone Cal"
                n688 = flat-sequence {
                  tunnel: w222 -> [w228]
                  tunnel: [w228] -> w221
                  frame #0 {
                    w227 = u16 0 ("Mic Type")
                    w229 = u16 0 ("Signal Type In")
                    n689 = global write "CRYCal Global.vi" "Signal Type In"(w229) -> ()
                    n690 = global write "CRYCal Global.vi" "Signal Type Out"(w229) -> ()
                    n691 = global write "CRYCal Global.vi" "Calibrator Type"(w227) -> ()
                    n692 = global write "CRYCal Global.vi" "Mic Type"(w227) -> ()
                  }
                }
                n693 = call "CRYMicrophone Calibration.vi"("Hardware in"=w226, "Old Total Sens"=w221) -> ("Ref. Freq out"=w220:dbl, "Completed"=w224:bool, "Total Sens"=w225:dbl)  [unwired: 3 in, 4 out]
                n694 = Not(x=w224) -> (.not. x?=w223:bool)
              }
            }
          }
          frame #1 {
            n695 = case shown="False" w269 {
              tunnel: w271 -> [w272 _]
              tunnel: w270 -> [w275 _]
              tunnel: w269 -> [_ _]
              frame False {
                n696 = local read "Calibration"() -> (w277:T1)
                n697 = property on="Input Signal Type" class="Ring (strict)"() -> ("RingText.Text"=w274:string)  [unwired: 2 in, 2 out]
                n698 = Build Array(w274) -> (w279:string[])
                n699 = local write "Sensitivity In"(w272) -> ()
                n700 = Unbundle By Name(w277) -> ("Calibration 2D"=w282:T2[])
                n701 = call "CRYGet Channel From Signal Type.vi"("Calibration"=w277, "Signal Type Name Array In"=w279, "In/Out?"=TRUE) -> ("equal Index Out"=w276:i32[])  [unwired: 7 in, 1 out]
                n702 = Index Array(array=w276) -> (element=w273:i32)  [unwired: 1 in]
                n703 = local write "Signal Type Index"(w273) -> ()
                n704 = Index Array(array=w282, index=w273) -> (element=w287:T2)
                n705 = Unbundle By Name(w287) -> ("Sens Curve.Curve"=w286:cluster{"x":dbl, "y":dbl, "z":dbl}[])
                n706 = local write "Hz In"(w275) -> ()
                n707 = call "CRYConversion dB-Lin.vi"("dB ref."=1.0, "Lin In"=w272) -> ("Log Out"=w291:dbl)  [unwired: 4 in, 3 out]
                n708 = local write "dB In"(w291) -> ()
                n709 = Index Array(array=w286, index=0) -> (element=w284:cluster{"x":dbl, "y":dbl, "z":dbl})
                n710 = Bundle By Name(cluster=w284, "x"=w275, "y"=w272) -> (w290:cluster{"x":dbl, "y":dbl, "z":dbl})
                n711 = Build Array(w290) -> (w289:cluster{"x":dbl, "y":dbl, "z":dbl}[])
                n712 = Bundle By Name(cluster=w287, "Sens Curve.Curve"=w289) -> (w288:T2)
                n713 = Replace Array Subset(array=w282, new element=w288, index=w273) -> (w281:T2[])
                n714 = Bundle By Name(cluster=w277, "Calibration 2D"=w281) -> (w280:T1)
                n715 = local write "Calibration"(w280) -> ()
              }
              frame True {
              }
            }
          }
          frame #2 {
            n716 = Not(x=w293) -> (.not. x?=w292:bool)
            n717 = global write "CRYCal Global.vi" "Calibrate"(FALSE ("Calibrate")) -> ()
            n718 = local write "Insert flag"(w292) -> ()
          }
        }
      }
      frame 3 {
        n719 = local read "dB ref Out"() -> (w300:dbl)
        n720 = local read "unit Out"() -> (w301:string)
        n721 = call "CRYUnits setup.vi"("Scale visible?"=FALSE, "dB/Lin"=u16 0 ("Scale"), "Unit:"=w301, "dB ref:"=w300, "Custom unit settings"=T7 {"Custom units dialog?"=FALSE, "Use custom unit?"=FALSE}, "Common dB ref."=u16 0) -> ("New unit Lin"=w303:string, "New dB ref"=w302:dbl, "Cancelled?"=w296:bool)  [unwired: 2 in, 5 out]
        n722 = case shown="False" w296 {
          tunnel: w303 -> [w305 _]
          tunnel: w302 -> [w304 _]
          frame False {
            n723 = local write "dB ref Out"(w304) -> ()
            n724 = local write "unit Out"(w305) -> ()
            n725 = flat-sequence {
              tunnel: w305 -> [w326]
              tunnel: w304 -> [w325]
              frame #0 {
                n726 = local read "Calibration"() -> (w318:T1)
                n727 = property on="Output Signal Type" class="Ring (strict)"() -> ("RingText.Text"=w307:string)  [unwired: 2 in, 2 out]
                n728 = call "CRYGet IOCalibration 2D.vi"("Calibration"=w318) -> ("O_Calibration 2D Out"=w314:T2[], "I_Calibration 2D Out"=w317:T2[])  [unwired: 9 in]
                n729 = call "CRYGet Cal Info From SignalType and Channel Name.vi"("Signal Type"=w307, "In/Out?"=FALSE) -> ("Index"=w306:i32)  [unwired: 7 in, 2 out]
                n730 = call "CRYGet Calibration 2D From Signal Type.vi"("I/O Calibration 2D"=w314, "Signal Type Name In"=w307) -> ("equal Index Out"=w313:i32)  [unwired: 8 in, 1 out]
                n731 = Index Array(array=w314, index=w313) -> (element=w323:T2)
                n732 = Unbundle By Name(w323) -> ("Sens Curve.Y unit"=w312:string)
                n733 = local write "Signal Type Index"(w306) -> ()
                n734 = Reverse String(1:w312) -> (0:w311:string)
                n735 = Match Pattern(string=w311, regular expression="/") -> (before substring=w309:string, match substring=w321:string)  [unwired: 1 in, 2 out]
                n736 = Reverse String(1:w309) -> (0:w310:string)
                n737 = Concatenate Strings(w326, w321, w310) -> (w320:string)
                n738 = Bundle By Name(cluster=w323, "Sens Curve.Y dB ref"=w325, "Sens Curve.Y unit"=w320) -> (w324:T2)
                n739 = local write "Sens unit Out"(w320) -> ()
                n740 = Replace Array Subset(array=w314, new element=w324, index=w313) -> (w316:T2[])
                n741 = Build Array (concatenate)(w316, w317) -> (w315:T2[])
                n742 = Bundle By Name(cluster=w318, "Calibration 2D"=w315) -> (w319:T1)
                n743 = local write "Calibration"(w319) -> ()
              }
              frame #1 {
                n744 = local write "Insert flag"(TRUE ("Insert flag")) -> ()
              }
            }
          }
          frame True {
          }
        }
      }
      frame 4 {
        n745 = flat-sequence {
          tunnel: [w345] -> w328
          tunnel: w328 -> [w370]
          frame #0 {
            w358 = u16 0 ("Signal Type In")
            n746 = local read "Hardware In"() -> (w352:string)
            n747 = property on="Output Signal Type" class="Ring (strict)"() -> ("RingText.Text"=w342:string)  [unwired: 2 in, 2 out]
            n748 = local read "Calibration"() -> (w348:T1)
            n749 = property on="Input Signal Type" class="Ring (strict)"() -> ("RingText.Text"=w337:string)  [unwired: 2 in, 2 out]
            n750 = property on="Channel Out" class="Ring (strict)"() -> ("Value"=w355:i32)  [unwired: 2 in, 2 out]
            n751 = Equal?(x=w342, y="Mouth Sim 1" ("EventName")) -> (x = y?=w341:bool)
            n752 = Equal?(x=w342, y="Mouth Sim 2" ("EventName")) -> (x = y?=w340:bool)
            n753 = call "CRYGet Hardware IO Infor.vi"("Hardware setup In"=w352) -> ("I_channel Info Out"=w354:T12[], "O_channel Info Out"=w353:T12[])  [unwired: 9 out]
            n754 = Build Array(w342) -> (w361:string[])
            n755 = Or(x=w341, y=w340) -> (x .or. y?=w339:bool)
            n756 = Index Array(array=w353, index=w355) -> (element=w356:T12)
            n757 = Select(t="Mic 1" ("EventName"), s=w339, f=w337) -> (s? t:f=w336:string)
            n758 = global write "CRYCal Global.vi" "Output Hardware Cal"(w356) -> ()
            n759 = global write "CRYCal Global.vi" "Sens Out"(1.0 ("Sens Out")) -> ()
            n760 = call "CRYGet Cal Info From SignalType and Channel Name.vi"("Calibration"=w348, "Signal Type"=w336, "In/Out?"=TRUE) -> ("Calibration 2D Cluster"=w332:T2)  [unwired: 6 in, 2 out]
            n761 = call "CRYGet Cal Info From SignalType and Channel Name.vi"("Calibration"=w348, "Signal Type"=w342, "In/Out?"=FALSE) -> ("Calibration 2D Cluster"=w346:T2)  [unwired: 6 in, 2 out]
            n762 = call "CRYGet Channel From Signal Type.vi"("Calibration"=w348, "Signal Type Name Array In"=w361, "In/Out?"=FALSE) -> ("equal Index Out"=w362:i32[])  [unwired: 7 in, 1 out]
            n763 = property on="Channel In" class="Ring (strict)"() -> ("Strings []"=w335:string[])  [unwired: 2 in, 2 out]
            n764 = Unbundle By Name(w332) -> ("Calibration.Cha Name"=w334:string)
            n765 = Unbundle By Name(w332) -> ("Sens Curve.Curve"=w330:cluster{"x":dbl, "y":dbl, "z":dbl}[])
            n766 = Index Array(array=w362) -> (element=w345:i32)  [unwired: 1 in]
            n767 = global write "CRYCal Global.vi" "Output Cal"(w346) -> ()
            n768 = global write "CRYCal Global.vi" "Input Cal"(w332) -> ()
            n769 = local write "Signal Type Index"(w345) -> ()
            n770 = global write "CRYCal Global.vi" "Calibration Calibrate"(TRUE ("Calibration Calibrate")) -> ()
            n771 = global write "CRYCal Global.vi" "Signal Type In"(w358) -> ()
            n772 = global write "CRYCal Global.vi" "Signal Type Out"(w358) -> ()
            n773 = global write "CRYCal Global.vi" "Calibrate"(TRUE ("Calibrate")) -> ()
            n774 = Search 1D Array(1D array=w335, element=w334) -> (index of element=w333:i32)  [unwired: 1 in]
            n775 = Index Array(array=w354, index=w333) -> (element=w357:T12)
            n776 = global write "CRYCal Global.vi" "Input Hardware Cal"(w357) -> ()
            n777 = call "CRYBackup Work State.vi"() -> ()  [unwired: 12 in]
            n778 = Index Array(array=w330) -> (element=w331:cluster{"x":dbl, "y":dbl, "z":dbl})  [unwired: 1 in]
            n779 = Unbundle By Name(w331) -> ("y"=w329:dbl)
            n780 = global write "CRYCal Global.vi" "Sens In"(w329) -> ()
          }
          frame #1 {
            n781 = property on="CalibrationSeq Out" class="Ring (strict)"() -> ("RingText.Text"=w367:string)  [unwired: 2 in, 2 out]
            n782 = call "CRYRun Selected Project.vi"("sequence name"=w367) -> ("run state"=w371:bool)  [unwired: 10 out]
            n783 = Equal?(x=w367, y="Direct Calibration" ("EventName")) -> (x = y?=w365:bool)
            n784 = Equal?(x=w367, y="Amplifier Calibration" ("EventName")) -> (x = y?=w366:bool)
            n785 = Or(x=w366, y=w365) -> (x .or. y?=w364:bool)
            n786 = call "CRYGet Current TS Steps.vi"() -> ("Steps"=w363:T6[])  [unwired: 7 in, 4 out]
            n787 = case shown="False" w364 {
              tunnel: w370 -> [w374 w421]
              tunnel: w371 -> [w373 w420]
              tunnel: w363 -> [w372 w419]
              frame True {
                # "Amp Cal & Direct Cal"
                n788 = case shown="True" w373 {
                  tunnel: w374 -> [_ w382]
                  tunnel: w372 -> [_ w380]
                  frame False {
                  }
                  frame True {
                    n789 = local read "Calibration"() -> (w384:T1)
                    n790 = Unbundle By Name(w384) -> ("Calibration 2D"=w383:T2[])
                    n791 = call "CRYGet Curve Library Array.vi"("Type In"=enum16{"Curves", "Values", "Results", "WFM"}."Curves") -> ("Curve/Value array"=w377:T17)  [unwired: 8 in, 2 out]
                    n792 = call "CRYGet Curve Library Array.vi"("Type In"=enum16{"Curves", "Values", "Results", "WFM"}."Values") -> ("Curve/Value array"=w376:T17)  [unwired: 8 in, 2 out]
                    n793 = Build Array (concatenate)(w377, w376) -> (w375:T17)
                    n794 = Index Array(array=w383, index=w382) -> (element=w381:T2)
                    n795 = call "CRYGet Curve & Sensitiviy.vi"("Calibration Cluster"=w381, "Finished test? (T)"=TRUE ("Calibrate? (F)"), "Data stack out"=w375) -> ("Success?"=w385:bool, "Sensitivity"=w388:dbl, "corr-out curve"=w387:cluster{"x":dbl, "y":dbl, "z":dbl}[], "eq- out curve"=w389:cluster{"x":dbl, "y":dbl, "z":dbl}[])  [unwired: 3 in, 2 out]
                    n796 = case shown="True" w385 {
                      tunnel: w389 -> [_ w393]
                      tunnel: w388 -> [_ w397]
                      tunnel: w382 -> [_ w409]
                      tunnel: w387 -> [_ w392]
                      tunnel: w384 -> [_ w396]
                      tunnel: w383 -> [_ w395]
                      tunnel: w381 -> [_ w394]
                      tunnel: w380 -> [_ w391]
                      frame False {
                      }
                      frame True {
                        # "???????"
                        n797 = for {
                          tunnel: w391 -> [w418] mode=indexing
                          tunnel: [w417] -> w405 mode=indexing
                          n798 = Unbundle By Name(w418) -> ("Category"=w417:string)
                        }
                        n799 = Unbundle By Name(w394) -> ("Sens Curve.Curve"=w416:cluster{"x":dbl, "y":dbl, "z":dbl}[])
                        n800 = Search 1D Array(1D array=w405, element="Stimulus" ("Category name")) -> (index of element=w403:i32)  [unwired: 1 out]
                        n801 = Index Array(array=w391, index=w403) -> (element=w402:T6)
                        n802 = Unbundle By Name(w402) -> ("Seq setup flattened"=w401:string)
                        n803 = call "CRYUnflatten Stimulus.vi"("Flatten Stimulus"=w401) -> ("Stimulus"=w408:T18)  [unwired: 10 out]
                        n804 = Unbundle By Name(w408) -> ("StepResolutionArray"=w407:u16[])
                        n805 = Index Array(array=w416, index=0) -> (element=w414:cluster{"x":dbl, "y":dbl, "z":dbl})
                        n806 = Bundle By Name(cluster=w414, "y"=w397) -> (w413:cluster{"x":dbl, "y":dbl, "z":dbl})
                        n807 = local write "Sensitivity Out"(w397) -> ()
                        n808 = Build Array(w413) -> (w412:cluster{"x":dbl, "y":dbl, "z":dbl}[])
                        n809 = Index Array(array=w407, index=0) -> (element=w399:u16)
                        n810 = Bundle By Name(cluster=w394, "EQ Curve.Curve"=w393, "Corr Curve.Curve"=w392, "Sens Curve.Curve"=w412, "Calibration.Corr Step size"=w399) -> (w410:T2)
                        n811 = call "CRYConversion dB-Lin.vi"("dB ref."=1.0, "Lin In"=w397) -> ("Log Out"=w411:dbl)  [unwired: 4 in, 3 out]
                        n812 = local write "dB Out"(w411) -> ()
                        n813 = Replace Array Subset(array=w395, new element=w410, index=w409) -> (w398:T2[])
                        n814 = Bundle By Name(cluster=w396, "Calibration 2D"=w398) -> (w390:T1)
                        n815 = local write "Calibration"(w390) -> ()
                      }
                    }
                  }
                }
              }
              frame False {
                # "Anechoic Test Box Cal & Mouth Cal & Anechoic Room Cal & Simulated Free Field Cal"
                n816 = case shown="True" w420 {
                  tunnel: w421 -> [_ w430]
                  tunnel: w419 -> [_ w427]
                  frame False {
                  }
                  frame True {
                    n817 = local read "Calibration"() -> (w431:T1)
                    n818 = call "CRYGet Curve Library Array.vi"("Type In"=enum16{"Curves", "Values", "Results", "WFM"}."Curves") -> ("Curve/Value array"=w425:T17)  [unwired: 8 in, 2 out]
                    n819 = call "CRYGet Curve Library Array.vi"("Type In"=enum16{"Curves", "Values", "Results", "WFM"}."Values") -> ("Curve/Value array"=w426:T17)  [unwired: 8 in, 2 out]
                    n820 = Unbundle By Name(w431) -> ("Calibration 2D"=w429:T2[])
                    n821 = Build Array (concatenate)(w425, w426) -> (w422:T17)
                    n822 = Index Array(array=w429, index=w430) -> (element=w428:T2)
                    n823 = call "CRYGet Curve & Sensitiviy.vi"("Calibration Cluster"=w428, "Finished test? (T)"=TRUE ("Calibrate? (F)"), "Data stack out"=w422) -> ("Success?"=w436:bool, "Sensitivity"=w435:dbl, "corr-out curve"=w432:cluster{"x":dbl, "y":dbl, "z":dbl}[], "eq- out curve"=w433:cluster{"x":dbl, "y":dbl, "z":dbl}[])  [unwired: 2 in, 3 out]
                    n824 = case shown="True" w436 {
                      tunnel: w433 -> [_ w444]
                      tunnel: w435 -> [_ w448]
                      tunnel: w430 -> [_ w456]
                      tunnel: w432 -> [_ w443]
                      tunnel: w431 -> [_ w442]
                      tunnel: w429 -> [_ w441]
                      tunnel: w428 -> [_ w440]
                      tunnel: w427 -> [_ w439]
                      frame False {
                      }
                      frame True {
                        # "?????????"
                        n825 = for {
                          tunnel: w439 -> [w465] mode=indexing
                          tunnel: [w464] -> w452 mode=indexing
                          n826 = Unbundle By Name(w465) -> ("Category"=w464:string)
                        }
                        n827 = Unbundle By Name(w440) -> ("Sens Curve.Curve"=w463:cluster{"x":dbl, "y":dbl, "z":dbl}[])
                        n828 = Search 1D Array(1D array=w452, element="Stimulus" ("Category name")) -> (index of element=w451:i32)  [unwired: 1 out]
                        n829 = Index Array(array=w439, index=w451) -> (element=w450:T6)
                        n830 = Unbundle By Name(w450) -> ("Seq setup flattened"=w449:string)
                        n831 = call "CRYUnflatten Stimulus.vi"("Flatten Stimulus"=w449) -> ("Stimulus"=w455:T18)  [unwired: 10 out]
                        n832 = Unbundle By Name(w455) -> ("StepResolutionArray"=w454:u16[])
                        n833 = Index Array(array=w463, index=0) -> (element=w461:cluster{"x":dbl, "y":dbl, "z":dbl})
                        n834 = local write "Sensitivity Out"(w448) -> ()
                        n835 = Bundle By Name(cluster=w461, "y"=w448) -> (w460:cluster{"x":dbl, "y":dbl, "z":dbl})
                        n836 = Build Array(w460) -> (w459:cluster{"x":dbl, "y":dbl, "z":dbl}[])
                        n837 = Index Array(array=w454, index=0) -> (element=w446:u16)
                        n838 = Bundle By Name(cluster=w440, "EQ Curve.Curve"=w444, "Corr Curve.Curve"=w443, "Sens Curve.Curve"=w459, "Calibration.Corr Step size"=w446, "Calibration.EQ Step size"=w446) -> (w457:T2)
                        n839 = call "CRYConversion dB-Lin.vi"("dB ref."=1.0, "Lin In"=w448) -> ("Log Out"=w458:dbl)  [unwired: 4 in, 3 out]
                        n840 = local write "dB Out"(w458) -> ()
                        n841 = Replace Array Subset(array=w441, new element=w457, index=w456) -> (w445:T2[])
                        n842 = Bundle By Name(cluster=w442, "Calibration 2D"=w445) -> (w437:T1)
                        n843 = local write "Calibration"(w437) -> ()
                      }
                    }
                  }
                }
              }
            }
          }
          frame #2 {
            n844 = call "CRYRestore Work State.vi"() -> ()  [unwired: 12 in]
            n845 = call "CRYBackup All.vi"("sOption"="Restore") -> ()  [unwired: 11 in]
          }
          frame #3 {
            n846 = global write "CRYCal Global.vi" "Calibration Calibrate"(FALSE ("Calibration Calibrate")) -> ()
            n847 = local write "Insert flag"(TRUE ("Insert flag")) -> ()
            n848 = global write "CRYCal Global.vi" "Calibrate"(FALSE ("Calibrate")) -> ()
          }
        }
      }
      frame 5 {
        n849 = case shown="True" w470 {
          frame False {
          }
          frame True {
            n850 = local read "Calibration"() -> (w472:T1)
            n851 = Unbundle By Name(w472) -> ("Calibration 2D"=w471:T2[])
            n852 = call "CRYSignal Path Table.vi"("Calibration"=w471) -> ()  [unwired: 11 in]
          }
        }
      }
      frame 6 {
        n853 = local read "Calibration"() -> (w476:T1)
        n854 = local write "Insert flag"(FALSE ("Insert flag")) -> ()
        n855 = local read "Signal Type Index"() -> (w474:i32)
        n856 = Unbundle By Name(w476) -> ("Calibration 2D"=w477:T2[])
        n857 = Index Array(array=w477, index=w474) -> (element=w478:T2)
        n858 = for {
          tunnel: w477 -> [w483] mode=indexing
          tunnel: w478 -> [w481]
          tunnel: [w482] -> w475 mode=indexing
          tunnel: w474 -> [w480]
          i -> [w489]
          n859 = Unbundle By Name(w483) -> ("Calibration.Calibrated Device"=w488:string)
          n860 = Unbundle By Name(w481) -> ("Calibration.Calibrated Device"=w487:string)
          n861 = Not Equal?(x=w480, y=w489) -> (x != y?=w485:bool)
          n862 = Equal?(x=w488, y=w487) -> (x = y?=w486:bool)
          n863 = And(x=w486, y=w485) -> (x .and. y?=w484:bool)
          n864 = case shown="True" w484 {
            tunnel: [w490 w493] -> w482
            tunnel: w483 -> [w490 w496]
            tunnel: w481 -> [_ w495]
            frame False {
            }
            frame True {
              n865 = Unbundle By Name(w496) -> ("Calibration.Signal Type"=w494:string, "Calibration.Cha Name"=w492:string, "Calibration.Device"=w491:string)
              n866 = Bundle By Name(cluster=w495, "Calibration.Signal Type"=w494, "Calibration.Cha Name"=w492, "Calibration.Device"=w491) -> (w493:T2)
            }
          }
        }
        n867 = Bundle By Name(cluster=w476, "Calibration 2D"=w475) -> (w473:T1)
        n868 = local write "Calibration"(w473) -> ()
      }
      frame 7 {
        n869 = flat-sequence {
          frame #0 {
            n870 = global read "CRYProject Editor Global.vi" "Calibration Step"() -> (w497:T6)
            n871 = local read "Calibration"() -> (w504:T1)
            n872 = local write "Cal_ValueChange"(FALSE ("Cal_ValueChange")) -> ()
            n873 = Unbundle By Name(w497) -> ("Seq setup flattened"=w506:string)
            n874 = Unbundle By Name(w504) -> ("Tab Value"=w501:i32, "Input Signal Type"=w500:string, "Output Signal Type"=w499:string, "Help"=w498:string)
            n875 = call "CRYUnflatten Calibration 2D.vi"("Flattened Calibration"=w506) -> ("Calibration Step Out"=w503:T1)  [unwired: 2 in, 8 out]
            n876 = Bundle By Name(cluster=w503, "Tab Value"=w501, "Input Signal Type"=w500, "Output Signal Type"=w499, "Help"=w498) -> (w502:T1)
            n877 = local write "Calibration"(w502) -> ()
          }
          frame #1 {
            n878 = local write "Load Test"(TRUE ("Cal_ValueChange")) -> ()
          }
        }
      }
      frame 8..15 {
        # "I_Add/Delete/Rename/Copy"
        n879 = Subtract(x=w520, y=8) -> (x-y=w511:i32)
        n880 = call "CRYGet Error Message.vi"("Error No"=0, "Kind"="Calibration Sub") -> ("Message Sub"=w518:string[])  [unwired: 4 in, 5 out]
        n881 = Quotient & Remainder(x=w511, y=4) -> (x-y*floor(x/y)=w510:i32, floor(x/y)=w514:i32)
        n882 = Index Array(array=w518, index=w510) -> (element=w521:string)
        n883 = case shown="1, Default" w514 {
          tunnel: [w689 w692] -> w512
          tunnel: ["Output Calibration Data" ("name or relative path") "Input Calibration Data" ("name or relative path")] -> w516
          tunnel: [FALSE ("Input/Output") TRUE ("Input/Output")] -> w508
          frame 1, Default {
            n884 = property on="Calibrated Output Device" class="Ring (strict)"() -> ("RingText.Text"=w689:string)  [unwired: 2 in, 2 out]
          }
          frame 0 {
            n885 = property on="Calibrated Input Device" class="Ring (strict)"() -> ("RingText.Text"=w692:string)  [unwired: 2 in, 2 out]
          }
        }
        n886 = case shown="0" w510 {
          tunnel: [w698 w702 w714 w724] -> w517
          tunnel: w521 -> [w693 _ w713 w723]
          tunnel: [w694 w699 w712 w722] -> w515
          tunnel: w512 -> [_ w699 w708 w716]
          frame 0 {
            # "Add"
            n887 = call "CRYGet Channel Name Dialog.vi"("Channel Name"="", "Window Title"=w693) -> ("Channel Name Out"=w695:string, "Return Flag"=w698:bool)  [unwired: 8 out]
            n888 = Concatenate Strings(w695, ".dat" ("string")) -> (w694:string)
          }
          frame 1 {
            # "Delete"
            n889 = call "CRYGet Error Message.vi"("Error No"=4 ("No"), "Kind"="Calibration") -> ("Message"=w704:string, "Window Title"=w700:string)  [unwired: 4 in, 4 out]
            n890 = Format Into String(format string=w704, w699) -> (resulting string=w703:string)  [unwired: 2 in, 1 out]
            n891 = call "CRYMessage Dialog.vi"("Window Title"=w700, "YesNoCancel"=T8."YesNo", "Message Content"=w703) -> ("YesNo"=w702:bool)  [unwired: 7 in, 1 out]
          }
          frame 2 {
            # "Rename"
            n892 = Reverse String(1:w708) -> (0:w710:string)
            n893 = Match Pattern(string=w710, regular expression="[.]") -> (after substring=w711:string)  [unwired: 4 out]
            n894 = Reverse String(1:w711) -> (0:w707:string)
            n895 = call "CRYGet Channel Name Dialog.vi"("Channel Name"=w707, "Window Title"=w713) -> ("Channel Name Out"=w712:string, "Return Flag"=w714:bool)  [unwired: 8 out]
          }
          frame 3, Default {
            # "Copy"
            n896 = Reverse String(1:w716) -> (0:w718:string)
            n897 = Match Pattern(string=w718, regular expression="[.]") -> (after substring=w719:string)  [unwired: 4 out]
            n898 = Reverse String(1:w719) -> (0:w715:string)
            n899 = Concatenate Strings("Copy of " ("RingText.Text"), w715) -> (w720:string)
            n900 = call "CRYGet Channel Name Dialog.vi"("Channel Name"=w720, "Window Title"=w723) -> ("Channel Name Out"=w722:string, "Return Flag"=w724:bool)  [unwired: 8 out]
          }
        }
        n901 = Equal To 0?(x=w514) -> (x = 0?=w513:bool)
        n902 = case shown="True" w517 {
          tunnel: w510 -> [_ w529]
          tunnel: w516 -> [_ w528]
          tunnel: w515 -> [_ w527]
          tunnel: w513 -> [_ w526]
          tunnel: w512 -> [_ w525]
          tunnel: w508 -> [_ w524]
          frame False {
          }
          frame True {
            n903 = case shown="1" w529 {
              tunnel: w528 -> [w536 w573 w608 w644]
              tunnel: w527 -> [w531 w572 w607 w646]
              tunnel: w526 -> [w535 w575 w610 w645]
              tunnel: w525 -> [_ _ w616 _]
              tunnel: w524 -> [_ w571 _ _]
              frame 0 {
                # "Add"
                n904 = local read "Calibration"() -> (w534:T1)
                n905 = global read "CRYMainGlobal.vi" "Calibration path"() -> (w540:path)
                n906 = property on="Channel Out" class="Ring (strict)"() -> ("Value"=w541:i32)  [unwired: 2 in, 2 out]
                n907 = property on="Channel Out" class="Ring (strict)"() -> ("Strings []"=w546:string[])  [unwired: 2 in, 2 out]
                n908 = property on="Channel In" class="Ring (strict)"() -> ("Value"=w547:i32)  [unwired: 2 in, 2 out]
                n909 = Array Size(array=w546) -> (size(s)=w545:i32)
                n910 = Concatenate Strings(w536, "\\" ("string"), w531) -> (w538:string)
                n911 = Unbundle By Name(w534) -> ("Calibration 2D"=w532:T2[])
                n912 = Add(x=w545, y=w547) -> (x+y=w542:i32)
                n913 = Build Path(base path=w540, name or relative path=w538) -> (appended path=w537:path)
                n914 = Select(t=w542, s=w535, f=w541) -> (s? t:f=w533:i32)
                n915 = Index Array(array=w532, index=w533) -> (element=w530:T2)
                n916 = call "CRYFlatten Calibration Data File.vi"("Calibration 2D Cluster"=w530) -> ("Calibration2D flattened"=w544:string)  [unwired: 10 in]
                n917 = call "CRYFlatten Data Save.vi"("Any Flatten Data"=w544, "Path In"=w537) -> ("error out"=w543:errorcluster)  [unwired: 6 in, 1 out]
                n918 = case shown="No Error" w543 {
                  tunnel: w535 -> [w552 _]
                  tunnel: w531 -> [w551 _]
                  tunnel: w536 -> [w549 _]
                  tunnel: w533 -> [_ _]
                  frame No Error {
                    n919 = global read "CRYMainGlobal.vi" "Calibration path"() -> (w553:path)
                    n920 = Build Path(base path=w553, name or relative path=w549) -> (appended path=w554:path)
                    n921 = List Folder(path=w554) -> (filenames=w548:string[])  [unwired: 3 in, 3 out]
                    n922 = Search 1D Array(1D array=w548, element=w551) -> (index of element=w550:i32)  [unwired: 1 in]
                    n923 = case shown="True" w552 {
                      tunnel: w548 -> [w557 w563]
                      tunnel: w550 -> [w556 w562]
                      frame False {
                        n924 = flat-sequence {
                          tunnel: w557 -> [w559]
                          tunnel: w556 -> [w558]
                          tunnel: [w558] -> w555
                          tunnel: w555 -> [w560]
                          frame #0 {
                            n925 = property on="Calibrated Output Device" class="Ring (strict)"("Strings []"=w559) -> ()  [unwired: 2 in, 2 out]
                          }
                          frame #1 {
                            n926 = property on="Calibrated Output Device" class="Ring (strict)"("Val(Sgnl)"=w560) -> ()  [unwired: 2 in, 2 out]
                          }
                        }
                      }
                      frame True {
                        n927 = flat-sequence {
                          tunnel: w563 -> [w565]
                          tunnel: w562 -> [w564]
                          tunnel: [w564] -> w561
                          tunnel: w561 -> [w566]
                          frame #0 {
                            n928 = property on="Calibrated Input Device" class="Ring (strict)"("Strings []"=w565) -> ()  [unwired: 2 in, 2 out]
                          }
                          frame #1 {
                            n929 = property on="Calibrated Input Device" class="Ring (strict)"("Val(Sgnl)"=w566) -> ()  [unwired: 2 in, 2 out]
                          }
                        }
                      }
                    }
                  }
                  frame Error {
                    # "File Save Error"
                    n930 = call "CRYGet Error Message.vi"("Error No"=5 ("No"), "Kind"="Calibration") -> ("Message"=w567:string, "Window Title"=w570:string)  [unwired: 4 in, 4 out]
                    n931 = call "CRYMessage Dialog.vi"("Window Title"=w570, "Message Content"=w567) -> ()  [unwired: 8 in, 2 out]
                  }
                }
              }
              frame 1 {
                # "Delete"
                n932 = global read "CRYMainGlobal.vi" "Calibration path"() -> (w579:path)
                n933 = Concatenate Strings(w573, "\\" ("string"), w572) -> (w577:string)
                n934 = Build Path(base path=w579, name or relative path=w577) -> (appended path=w576:path)
                n935 = Delete(path (use dialog)=w576) -> (error out=w574:errorcluster)  [unwired: 4 in, 2 out]
                n936 = case shown="No Error" w574 {
                  tunnel: w575 -> [w584 _]
                  tunnel: w573 -> [w582 _]
                  tunnel: w572 -> [w580 _]
                  tunnel: w571 -> [w581 _]
                  frame No Error {
                    n937 = global read "CRYMainGlobal.vi" "Calibration path"() -> (w585:path)
                    n938 = Build Path(base path=w585, name or relative path=w582) -> (appended path=w586:path)
                    n939 = List Folder(path=w586) -> (filenames=w583:string[])  [unwired: 3 in, 3 out]
                    n940 = case shown="True" w584 {
                      tunnel: w583 -> [w587 w593]
                      tunnel: w581 -> [_ w592]
                      tunnel: w580 -> [_ w590]
                      frame False {
                        n941 = flat-sequence {
                          tunnel: w587 -> [w588]
                          frame #0 {
                            n942 = property on="Calibrated Output Device" class="Ring (strict)"("Strings []"=w588) -> ()  [unwired: 2 in, 2 out]
                          }
                          frame #1 {
                            n943 = property on="Calibrated Output Device" class="Ring (strict)"("Val(Sgnl)"=0) -> ()  [unwired: 2 in, 2 out]
                          }
                        }
                      }
                      frame True {
                        n944 = flat-sequence {
                          tunnel: w593 -> [w600]
                          tunnel: w592 -> [w597]
                          tunnel: [w595] -> w591
                          tunnel: w590 -> [w594]
                          tunnel: w591 -> [w601]
                          frame #0 {
                            n945 = property on="Calibrated Input Device" class="Ring (strict)"("Strings []"=w600) -> ()  [unwired: 2 in, 2 out]
                            n946 = local read "Calibration"() -> (w598:T1)
                            n947 = call "CRYSet Default Calibrate Device After Delete.vi"("Deleted Calibrated Device"=w594, "Input/Output"=w597, "Calibration In"=w598) -> ("unity cal Name"=w596:string, "Calibration Out"=w599:T1)  [unwired: 7 in]
                            n948 = local write "Calibration"(w599) -> ()
                            n949 = Search 1D Array(1D array=w600, element=w596) -> (index of element=w595:i32)  [unwired: 1 in]
                          }
                          frame #1 {
                            n950 = property on="Calibrated Input Device" class="Ring (strict)"("Val(Sgnl)"=w601) -> ()  [unwired: 2 in, 2 out]
                          }
                        }
                      }
                    }
                  }
                  frame Error {
                    n951 = call "CRYGet Error Message.vi"("Error No"=6 ("No"), "Kind"="Calibration") -> ("Message"=w602:string, "Window Title"=w605:string)  [unwired: 4 in, 4 out]
                    n952 = call "CRYMessage Dialog.vi"("Window Title"=w605, "Message Content"=w602) -> ()  [unwired: 8 in, 2 out]
                  }
                }
              }
              frame 2 {
                # "Old name"
                # "New name"
                # "Rename"
                n953 = global read "CRYMainGlobal.vi" "Calibration path"() -> (w615:path)
                n954 = Concatenate Strings(w607, ".dat" ("string")) -> (w606:string)
                n955 = Concatenate Strings(w608, "\\" ("string"), w616) -> (w618:string)
                n956 = Concatenate Strings(w608, "\\" ("string"), w606) -> (w619:string)
                n957 = Build Path(base path=w615, name or relative path=w618) -> (appended path=w614:path)
                n958 = Build Path(base path=w615, name or relative path=w619) -> (appended path=w613:path)
                n959 = Move(source path=w614, 9:TRUE ("overwrite (F)"), 10:w613) -> (error out=w611:errorcluster)  [unwired: 2 in, 2 out]
                n960 = case shown="No Error" w611 {
                  tunnel: w608 -> [w624 _]
                  tunnel: w610 -> [w623 _]
                  tunnel: w606 -> [w622 _]
                  frame No Error {
                    n961 = global read "CRYMainGlobal.vi" "Calibration path"() -> (w626:path)
                    n962 = Build Path(base path=w626, name or relative path=w624) -> (appended path=w627:path)
                    n963 = List Folder(path=w627) -> (filenames=w621:string[])  [unwired: 3 in, 3 out]
                    n964 = Search 1D Array(1D array=w621, element=w622) -> (index of element=w625:i32)  [unwired: 1 in]
                    n965 = case shown="True" w623 {
                      tunnel: w621 -> [w630 w636]
                      tunnel: w625 -> [w629 w635]
                      frame False {
                        n966 = flat-sequence {
                          tunnel: w630 -> [w632]
                          tunnel: w629 -> [w631]
                          tunnel: [w631] -> w628
                          tunnel: w628 -> [w633]
                          frame #0 {
                            n967 = property on="Calibrated Output Device" class="Ring (strict)"("Strings []"=w632) -> ()  [unwired: 2 in, 2 out]
                          }
                          frame #1 {
                            n968 = property on="Calibrated Output Device" class="Ring (strict)"("Val(Sgnl)"=w633) -> ()  [unwired: 2 in, 2 out]
                          }
                        }
                      }
                      frame True {
                        n969 = flat-sequence {
                          tunnel: w636 -> [w638]
                          tunnel: w635 -> [w637]
                          tunnel: [w637] -> w634
                          tunnel: w634 -> [w639]
                          frame #0 {
                            n970 = property on="Calibrated Input Device" class="Ring (strict)"("Strings []"=w638) -> ()  [unwired: 2 in, 2 out]
                          }
                          frame #1 {
                            n971 = property on="Calibrated Input Device" class="Ring (strict)"("Val(Sgnl)"=w639) -> ()  [unwired: 2 in, 2 out]
                          }
                        }
                      }
                    }
                  }
                  frame Error {
                    n972 = call "CRYGet Error Message.vi"("Error No"=7 ("No"), "Kind"="Calibration") -> ("Message"=w640:string, "Window Title"=w643:string)  [unwired: 4 in, 4 out]
                    n973 = call "CRYMessage Dialog.vi"("Window Title"=w643, "Message Content"=w640) -> ()  [unwired: 8 in, 2 out]
                  }
                }
              }
              frame 3, Default {
                # "Copy"
                n974 = local read "Calibration"() -> (w663:T1)
                n975 = global read "CRYMainGlobal.vi" "Calibration path"() -> (w652:path)
                n976 = property on="Channel Out" class="Ring (strict)"() -> ("Value"=w653:i32)  [unwired: 2 in, 2 out]
                n977 = property on="Channel Out" class="Ring (strict)"() -> ("Strings []"=w659:string[])  [unwired: 2 in, 2 out]
                n978 = property on="Channel In" class="Ring (strict)"() -> ("Value"=w660:i32)  [unwired: 2 in, 2 out]
                n979 = Concatenate Strings(w646, ".dat" ("string")) -> (w647:string)
                n980 = Array Size(array=w659) -> (size(s)=w658:i32)
                n981 = Concatenate Strings(w644, "\\" ("string"), w647) -> (w650:string)
                n982 = Unbundle By Name(w663) -> ("Calibration 2D"=w662:T2[])
                n983 = Add(x=w658, y=w660) -> (x+y=w654:i32)
                n984 = Build Path(base path=w652, name or relative path=w650) -> (appended path=w649:path)
                n985 = Select(t=w654, s=w645, f=w653) -> (s? t:f=w657:i32)
                n986 = Index Array(array=w662, index=w657) -> (element=w661:T2)
                n987 = call "CRYFlatten Calibration Data File.vi"("Calibration 2D Cluster"=w661) -> ("Calibration2D flattened"=w656:string)  [unwired: 10 in]
                n988 = call "CRYFlatten Data Save.vi"("Any Flatten Data"=w656, "Path In"=w649) -> ("error out"=w655:errorcluster)  [unwired: 6 in, 1 out]
                n989 = case shown="No Error" w655 {
                  tunnel: w645 -> [w668 _]
                  tunnel: w647 -> [w667 _]
                  tunnel: w644 -> [w665 _]
                  frame No Error {
                    n990 = global read "CRYMainGlobal.vi" "Calibration path"() -> (w669:path)
                    n991 = Build Path(base path=w669, name or relative path=w665) -> (appended path=w670:path)
                    n992 = List Folder(path=w670) -> (filenames=w664:string[])  [unwired: 3 in, 3 out]
                    n993 = Search 1D Array(1D array=w664, element=w667) -> (index of element=w666:i32)  [unwired: 1 in]
                    n994 = case shown="True" w668 {
                      tunnel: w664 -> [w673 w679]
                      tunnel: w666 -> [w672 w678]
                      frame False {
                        n995 = flat-sequence {
                          tunnel: w673 -> [w675]
                          tunnel: w672 -> [w674]
                          tunnel: [w674] -> w671
                          tunnel: w671 -> [w676]
                          frame #0 {
                            n996 = property on="Calibrated Output Device" class="Ring (strict)"("Strings []"=w675) -> ()  [unwired: 2 in, 2 out]
                          }
                          frame #1 {
                            n997 = property on="Calibrated Output Device" class="Ring (strict)"("Val(Sgnl)"=w676) -> ()  [unwired: 2 in, 2 out]
                          }
                        }
                      }
                      frame True {
                        n998 = flat-sequence {
                          tunnel: w679 -> [w681]
                          tunnel: w678 -> [w680]
                          tunnel: [w680] -> w677
                          tunnel: w677 -> [w682]
                          frame #0 {
                            n999 = property on="Calibrated Input Device" class="Ring (strict)"("Strings []"=w681) -> ()  [unwired: 2 in, 2 out]
                          }
                          frame #1 {
                            n1000 = property on="Calibrated Input Device" class="Ring (strict)"("Val(Sgnl)"=w682) -> ()  [unwired: 2 in, 2 out]
                          }
                        }
                      }
                    }
                  }
                  frame Error {
                    # "File Save Error"
                    n1001 = call "CRYGet Error Message.vi"("Error No"=5 ("No"), "Kind"="Calibration") -> ("Message"=w683:string, "Window Title"=w686:string)  [unwired: 4 in, 4 out]
                    n1002 = call "CRYMessage Dialog.vi"("Window Title"=w686, "Message Content"=w683) -> ()  [unwired: 8 in, 2 out]
                  }
                }
              }
            }
          }
        }
      }
      frame 16..23 {
        # "I_SAdd/SDelete/SRename/SCopy"
        n1003 = Subtract(x=w735, y=16) -> (x-y=w727:i32)
        n1004 = call "CRYGet Error Message.vi"("Error No"=1, "Kind"="Calibration Sub") -> ("Message Sub"=w733:string[])  [unwired: 4 in, 5 out]
        n1005 = Quotient & Remainder(x=w727, y=4) -> (x-y*floor(x/y)=w726:i32, floor(x/y)=w730:i32)
        n1006 = Index Array(array=w733, index=w726) -> (element=w736:string)
        n1007 = case shown="1, Default" w730 {
          tunnel: [w852 w853] -> w728
          frame 1, Default {
            n1008 = property on="Output Signal Type" class="Ring (strict)"() -> ("RingText.Text"=w852:string)  [unwired: 2 in, 2 out]
          }
          frame 0 {
            n1009 = property on="Input Signal Type" class="Ring (strict)"() -> ("RingText.Text"=w853:string)  [unwired: 2 in, 2 out]
          }
        }
        n1010 = case shown="1" w726 {
          tunnel: [w857 w861 w869 w875] -> w732
          tunnel: w736 -> [w855 _ w868 w874]
          tunnel: [w854 w858 w867 w873] -> w731
          tunnel: w728 -> [_ w858 w866 w870]
          frame 0 {
            # "Add"
            n1011 = call "CRYGet Channel Name Dialog.vi"("Channel Name"="", "Window Title"=w855) -> ("Channel Name Out"=w854:string, "Return Flag"=w857:bool)  [unwired: 8 out]
          }
          frame 1 {
            # "Delete"
            n1012 = call "CRYGet Error Message.vi"("Error No"=4 ("No"), "Kind"="Calibration") -> ("Message"=w863:string, "Window Title"=w859:string)  [unwired: 4 in, 4 out]
            n1013 = Format Into String(format string=w863, w858) -> (resulting string=w862:string)  [unwired: 2 in, 1 out]
            n1014 = call "CRYMessage Dialog.vi"("Window Title"=w859, "YesNoCancel"=T8."YesNo", "Message Content"=w862) -> ("YesNo"=w861:bool)  [unwired: 7 in, 1 out]
          }
          frame 2 {
            # "Rename"
            n1015 = call "CRYGet Channel Name Dialog.vi"("Channel Name"=w866, "Window Title"=w868) -> ("Channel Name Out"=w867:string, "Return Flag"=w869:bool)  [unwired: 8 out]
          }
          frame 3, Default {
            # "Copy"
            n1016 = Concatenate Strings("Copy of " ("RingText.Text"), w870) -> (w871:string)
            n1017 = call "CRYGet Channel Name Dialog.vi"("Channel Name"=w871, "Window Title"=w874) -> ("Channel Name Out"=w873:string, "Return Flag"=w875:bool)  [unwired: 8 out]
          }
        }
        n1018 = Equal To 0?(x=w730) -> (x = 0?=w729:bool)
        n1019 = case shown="True" w732 {
          tunnel: w726 -> [_ w742]
          tunnel: w731 -> [_ w741]
          tunnel: w729 -> [_ w740]
          tunnel: w728 -> [_ w739]
          frame False {
          }
          frame True {
            n1020 = case shown="1" w742 {
              tunnel: w741 -> [w749 w791 w818]
              tunnel: w740 -> [w743 w792 w811]
              tunnel: w739 -> [w744 _ w812]
              frame 0, 3 {
                # "Add, Copy"
                n1021 = local read "Calibration"() -> (w747:T1)
                n1022 = call "CRYGet Cal Info From SignalType and Channel Name.vi"("Calibration"=w747, "Signal Type"=w749, "In/Out?"=w743) -> ("Exist"=w748:bool)  [unwired: 6 in, 2 out]
                n1023 = call "CRYGet Cal Info From SignalType and Channel Name.vi"("Calibration"=w747, "Signal Type"=w744, "In/Out?"=w743) -> ("Calibration 2D Cluster"=w745:T2, "Exist"=w746:bool)  [unwired: 6 in, 1 out]
                n1024 = case shown="False" w748 {
                  tunnel: w743 -> [w757 _]
                  tunnel: w749 -> [w756 _]
                  tunnel: w746 -> [_ _]
                  tunnel: w745 -> [w765 _]
                  frame False {
                    n1025 = local read "Calibration"() -> (w768:T1)
                    n1026 = Bundle By Name(cluster=w765, "Calibration.Signal Type"=w756) -> (w753:T2)
                    n1027 = local read "Origine Calibration"() -> (w752:T1)
                    n1028 = Unbundle By Name(w768) -> ("Calibration 2D"=w767:T2[])
                    n1029 = Unbundle By Name(w752) -> ("Calibration 2D"=w754:T2[])
                    n1030 = Build Array (concatenate)(w767, w753) -> (w766:T2[])
                    n1031 = Build Array (concatenate)(w754, w753) -> (w751:T2[])
                    n1032 = Bundle By Name(cluster=w768, "Calibration 2D"=w766) -> (w755:T1)
                    n1033 = call "CRYGet IO Signal Type Name.vi"("Calibration"=w755) -> ("Output Signal Type  Name Out"=w763:string[], "Input Signal Type Name Out"=w764:string[])  [unwired: 9 in]
                    n1034 = case shown="True" w757 {
                      tunnel: w764 -> [_ w778]
                      tunnel: w763 -> [w773 _]
                      tunnel: w756 -> [w772 w777]
                      frame False {
                        n1035 = flat-sequence {
                          tunnel: w773 -> [w774]
                          tunnel: w771 -> [w775]
                          frame #0 {
                            n1036 = property on="Output Signal Type" class="Ring (strict)"("Strings []"=w774) -> ()  [unwired: 2 in, 2 out]
                          }
                          frame #1 {
                            n1037 = property on="Output Signal Type" class="Ring (strict)"("Val(Sgnl)"=w775) -> ()  [unwired: 2 in, 2 out]
                          }
                        }
                        n1038 = Search 1D Array(1D array=w773, element=w772) -> (index of element=w771:i32)  [unwired: 1 in]
                      }
                      frame True {
                        n1039 = flat-sequence {
                          tunnel: w778 -> [w779]
                          tunnel: w776 -> [w780]
                          frame #0 {
                            n1040 = property on="Input Signal Type" class="Ring (strict)"("Strings []"=w779) -> ()  [unwired: 2 in, 2 out]
                          }
                          frame #1 {
                            n1041 = property on="Input Signal Type" class="Ring (strict)"("Val(Sgnl)"=w780) -> ()  [unwired: 2 in, 2 out]
                          }
                        }
                        n1042 = Search 1D Array(1D array=w778, element=w777) -> (index of element=w776:i32)  [unwired: 1 in]
                      }
                    }
                    n1043 = Bundle By Name(cluster=w752, "Calibration 2D"=w751) -> (w750:T1)
                    n1044 = local write "Origine Calibration"(w750) -> ()
                    n1045 = local write "Calibration"(w755) -> ()
                    n1046 = property on="O_Signal Type Name" class="Arr (strict)"() -> ("Value"=w760:string[][])  [unwired: 2 in, 2 out]
                    n1047 = property on="I_Signal Type Name" class="Arr (strict)"() -> ("Value"=w761:string[][])  [unwired: 2 in, 2 out]
                    n1048 = Select(t=w761, s=w757, f=w760) -> (s? t:f=w759:string[][])
                    n1049 = call "CRYSet Channel Changing State.vi"("Name In"=w759, "New Channel Name"=w756, "Mode"=enum16{"Add", "Delete", "Rename", "Load/Revert"}."Add") -> ("Name Out"=w758:string[][])  [unwired: 8 in]
                    n1050 = case shown="False" w757 {
                      tunnel: w758 -> [w769 w770]
                      frame False {
                        n1051 = property on="O_Signal Type Name" class="Arr (strict)"("Value"=w769) -> ()  [unwired: 2 in, 2 out]
                      }
                      frame True {
                        n1052 = property on="I_Signal Type Name" class="Arr (strict)"("Value"=w770) -> ()  [unwired: 2 in, 2 out]
                      }
                    }
                  }
                  frame True {
                    n1053 = call "CRYGet Error Message.vi"("Error No"=8 ("No"), "Kind"="Calibration") -> ("Message"=w781:string, "Window Title"=w784:string)  [unwired: 4 in, 4 out]
                    n1054 = call "CRYMessage Dialog.vi"("Window Title"=w784, "Message Content"=w781) -> ()  [unwired: 8 in, 2 out]
                  }
                }
              }
              frame 1 {
                # "Delete"
                n1055 = local read "Calibration"() -> (w802:T1)
                n1056 = local read "Origine Calibration"() -> (w789:T1)
                n1057 = call "CRYGet Cal Info From SignalType and Channel Name.vi"("Calibration"=w802, "Signal Type"=w791, "In/Out?"=w792) -> ("Index"=w786:i32)  [unwired: 6 in, 2 out]
                n1058 = Unbundle By Name(w802) -> ("Calibration 2D"=w801:T2[])
                n1059 = Unbundle By Name(w789) -> ("Calibration 2D"=w787:T2[])
                n1060 = Delete From Array(array=w787, index=w786) -> (array with subset deleted=w785:T2[])  [unwired: 1 in, 1 out]
                n1061 = Delete From Array(array=w801, index=w786) -> (array with subset deleted=w800:T2[])  [unwired: 1 in, 1 out]
                n1062 = Bundle By Name(cluster=w802, "Calibration 2D"=w800) -> (w790:T1)
                n1063 = call "CRYGet IO Signal Type Name.vi"("Calibration"=w790) -> ("Output Signal Type  Name Out"=w799:string[], "Input Signal Type Name Out"=w798:string[])  [unwired: 9 in]
                n1064 = case shown="True" w792 {
                  tunnel: w798 -> [_ w808]
                  tunnel: w799 -> [w805 _]
                  frame False {
                    n1065 = flat-sequence {
                      tunnel: w805 -> [w806]
                      frame #0 {
                        n1066 = property on="Output Signal Type" class="Ring (strict)"("Strings []"=w806) -> ()  [unwired: 2 in, 2 out]
                      }
                      frame #1 {
                        n1067 = property on="Output Signal Type" class="Ring (strict)"("Val(Sgnl)"=0) -> ()  [unwired: 2 in, 2 out]
                      }
                    }
                  }
                  frame True {
                    n1068 = flat-sequence {
                      tunnel: w808 -> [w809]
                      frame #0 {
                        n1069 = property on="Input Signal Type" class="Ring (strict)"("Strings []"=w809) -> ()  [unwired: 2 in, 2 out]
                      }
                      frame #1 {
                        n1070 = property on="Input Signal Type" class="Ring (strict)"("Val(Sgnl)"=0) -> ()  [unwired: 2 in, 2 out]
                      }
                    }
                  }
                }
                n1071 = Bundle By Name(cluster=w789, "Calibration 2D"=w785) -> (w788:T1)
                n1072 = local write "Origine Calibration"(w788) -> ()
                n1073 = local write "Calibration"(w790) -> ()
                n1074 = property on="O_Signal Type Name" class="Arr (strict)"() -> ("Value"=w795:string[][])  [unwired: 2 in, 2 out]
                n1075 = property on="I_Signal Type Name" class="Arr (strict)"() -> ("Value"=w796:string[][])  [unwired: 2 in, 2 out]
                n1076 = Select(t=w796, s=w792, f=w795) -> (s? t:f=w794:string[][])
                n1077 = call "CRYSet Channel Changing State.vi"("Name In"=w794, "Old Channel Name"=w791, "Mode"=enum16{"Add", "Delete", "Rename", "Load/Revert"}."Delete") -> ("Name Out"=w793:string[][])  [unwired: 8 in]
                n1078 = case shown="False" w792 {
                  tunnel: w793 -> [w803 w804]
                  frame False {
                    n1079 = property on="O_Signal Type Name" class="Arr (strict)"("Value"=w803) -> ()  [unwired: 2 in, 2 out]
                  }
                  frame True {
                    n1080 = property on="I_Signal Type Name" class="Arr (strict)"("Value"=w804) -> ()  [unwired: 2 in, 2 out]
                  }
                }
              }
              frame 2, Default {
                # "Rename"
                n1081 = local read "Calibration"() -> (w816:T1)
                n1082 = call "CRYGet Cal Info From SignalType and Channel Name.vi"("Calibration"=w816, "Signal Type"=w818, "In/Out?"=w811) -> ("Exist"=w817:bool)  [unwired: 6 in, 2 out]
                n1083 = call "CRYGet Cal Info From SignalType and Channel Name.vi"("Calibration"=w816, "Signal Type"=w812, "In/Out?"=w811) -> ("Calibration 2D Cluster"=w814:T2, "Index"=w813:i32, "Exist"=w815:bool)  [unwired: 6 in]
                n1084 = case shown="False" w817 {
                  tunnel: w811 -> [w819 _]
                  tunnel: w818 -> [w821 _]
                  tunnel: w815 -> [_ _]
                  tunnel: w814 -> [w834 _]
                  tunnel: w813 -> [w827 _]
                  tunnel: w812 -> [w820 _]
                  frame False {
                    n1085 = local read "Calibration"() -> (w835:T1)
                    n1086 = Bundle By Name(cluster=w834, "Calibration.Signal Type"=w821) -> (w828:T2)
                    n1087 = Unbundle By Name(w835) -> ("Calibration 2D"=w830:T2[])
                    n1088 = Replace Array Subset(array=w830, new element=w828, index=w827) -> (w829:T2[])
                    n1089 = Bundle By Name(cluster=w835, "Calibration 2D"=w829) -> (w831:T1)
                    n1090 = call "CRYGet IO Signal Type Name.vi"("Calibration"=w831) -> ("Output Signal Type  Name Out"=w832:string[], "Input Signal Type Name Out"=w833:string[])  [unwired: 9 in]
                    n1091 = case shown="False" w819 {
                      tunnel: w833 -> [_ w845]
                      tunnel: w832 -> [w840 _]
                      tunnel: w821 -> [w839 w844]
                      frame False {
                        n1092 = flat-sequence {
                          tunnel: w840 -> [w841]
                          tunnel: w838 -> [w842]
                          frame #0 {
                            n1093 = property on="Output Signal Type" class="Ring (strict)"("Strings []"=w841) -> ()  [unwired: 2 in, 2 out]
                          }
                          frame #1 {
                            n1094 = property on="Output Signal Type" class="Ring (strict)"("Val(Sgnl)"=w842) -> ()  [unwired: 2 in, 2 out]
                          }
                        }
                        n1095 = Search 1D Array(1D array=w840, element=w839) -> (index of element=w838:i32)  [unwired: 1 in]
                      }
                      frame True {
                        n1096 = flat-sequence {
                          tunnel: w845 -> [w846]
                          tunnel: w843 -> [w847]
                          frame #0 {
                            n1097 = property on="Input Signal Type" class="Ring (strict)"("Strings []"=w846) -> ()  [unwired: 2 in, 2 out]
                          }
                          frame #1 {
                            n1098 = property on="Input Signal Type" class="Ring (strict)"("Val(Sgnl)"=w847) -> ()  [unwired: 2 in, 2 out]
                          }
                        }
                        n1099 = Search 1D Array(1D array=w845, element=w844) -> (index of element=w843:i32)  [unwired: 1 in]
                      }
                    }
                    n1100 = local write "Calibration"(w831) -> ()
                    n1101 = property on="I_Signal Type Name" class="Arr (strict)"() -> ("Value"=w825:string[][])  [unwired: 2 in, 2 out]
                    n1102 = property on="O_Signal Type Name" class="Arr (strict)"() -> ("Value"=w824:string[][])  [unwired: 2 in, 2 out]
                    n1103 = Select(t=w825, s=w819, f=w824) -> (s? t:f=w823:string[][])
                    n1104 = call "CRYSet Channel Changing State.vi"("Name In"=w823, "New Channel Name"=w821, "Old Channel Name"=w820, "Mode"=enum16{"Add", "Delete", "Rename", "Load/Revert"}."Rename") -> ("Name Out"=w822:string[][])  [unwired: 7 in]
                    n1105 = case shown="True" w819 {
                      tunnel: w822 -> [w836 w837]
                      frame False {
                        n1106 = property on="O_Signal Type Name" class="Arr (strict)"("Value"=w836) -> ()  [unwired: 2 in, 2 out]
                      }
                      frame True {
                        n1107 = property on="I_Signal Type Name" class="Arr (strict)"("Value"=w837) -> ()  [unwired: 2 in, 2 out]
                      }
                    }
                  }
                  frame True {
                    n1108 = call "CRYGet Error Message.vi"("Error No"=8 ("No"), "Kind"="Calibration") -> ("Message"=w848:string, "Window Title"=w851:string)  [unwired: 4 in, 4 out]
                    n1109 = call "CRYMessage Dialog.vi"("Window Title"=w851, "Message Content"=w848) -> ()  [unwired: 8 in, 2 out]
                  }
                }
              }
            }
          }
        }
      }
      frame 24, 25 {
        n1110 = Equal?(x=w887, y=24) -> (x = y?=w881:bool)
        n1111 = local read "Calibration"() -> (w877:T1)
        n1112 = property on="Input Signal Type" class="Ring (strict)"() -> ("RingText.Text"=w886:string)  [unwired: 2 in, 2 out]
        n1113 = property on="Output Signal Type" class="Ring (strict)"() -> ("RingText.Text"=w885:string)  [unwired: 2 in, 2 out]
        n1114 = Unbundle By Name(w877) -> ("Calibration 2D"=w882:T2[])
        n1115 = Select(t=w886, s=w881, f=w885) -> (s? t:f=w884:string)
        n1116 = call "CRYGet Cal Info From SignalType and Channel Name.vi"("Calibration"=w877, "Signal Type"=w884, "In/Out?"=w881) -> ("Index"=w876:i32)  [unwired: 6 in, 2 out]
        n1117 = Index Array(array=w882, index=w876) -> (element=w883:T2)
        n1118 = local write "Signal Type Index"(w876) -> ()
        n1119 = Unbundle By Name(w883) -> ("Calibration.Correction Curve Name"=w880:string, "Calibration.Equalization Curve Name"=w879:string)
        n1120 = case shown="True" w881 {
          tunnel: w880 -> [w895 w900]
          tunnel: w879 -> [w894 _]
          tunnel: [w893 w898] -> w878
          frame False {
            n1121 = call "CRYGet Curve Library Data.vi"("Type"=enum16{"Curves", "Values", "Results", "WFM"}."Curves", "Data Name"=w895) -> ("index"=w892:i32)  [unwired: 4 out]
            n1122 = call "CRYGet Curve Library Data.vi"("Type"=enum16{"Curves", "Values", "Results", "WFM"}."Curves", "Data Name"=w894) -> ("index"=w891:i32)  [unwired: 4 out]
            n1123 = Less Than 0?(x=w892) -> (x < 0?=w890:bool)
            n1124 = Less Than 0?(x=w891) -> (x < 0?=w889:bool)
            n1125 = Or(x=w890, y=w889) -> (x .or. y?=w893:bool)
          }
          frame True {
            n1126 = call "CRYGet Curve Library Data.vi"("Type"=enum16{"Curves", "Values", "Results", "WFM"}."Curves", "Data Name"=w900) -> ("index"=w899:i32)  [unwired: 4 out]
            n1127 = Less Than 0?(x=w899) -> (x < 0?=w898:bool)
          }
        }
        n1128 = case shown="False" w878 {
          tunnel: w879 -> [_ w912]
          tunnel: w880 -> [_ w911]
          tunnel: w881 -> [_ w910]
          tunnel: w877 -> [_ w906]
          tunnel: w876 -> [_ w909]
          frame True {
            n1129 = call "CRYGet Error Message.vi"("Error No"=12 ("No"), "Kind"="Calibration") -> ("Message"=w905:string, "Window Title"=w902:string)  [unwired: 4 in, 4 out]
            n1130 = call "CRYMessage Dialog.vi"("Window Title"=w902, "Message Content"=w905) -> ()  [unwired: 8 in, 2 out]
          }
          frame False, Default {
            n1131 = call "CRYImport Calibration Data Dialog.vi"("Invert Curve"=FALSE, "Index"=w909, "Calibration In"=w906, "EQ Name"=w912, "Corr Name"=w911, "In/Out Channel"=w910) -> ("Calibration Out"=w907:T1)  [unwired: 4 in, 1 out]
            n1132 = local write "Calibration"(w907) -> ()
            n1133 = flat-sequence {
              tunnel: w907 -> [w915]
              frame #0 {
                n1134 = property on="I_Signal Type Name" class="Arr (strict)"() -> ("Value"=w923:string[][])  [unwired: 2 in, 2 out]
                n1135 = property on="I_Calibrated Device Name" class="Arr (strict)"() -> ("Value"=w917:string[][])  [unwired: 2 in, 2 out]
                n1136 = property on="O_Calibrated Device Name" class="Arr (strict)"() -> ("Value"=w916:string[][])  [unwired: 2 in, 2 out]
                n1137 = property on="O_Signal Type Name" class="Arr (strict)"() -> ("Value"=w922:string[][])  [unwired: 2 in, 2 out]
                n1138 = local read "Proper VI No"() -> (w924:i32)
                n1139 = local read "Hardware In"() -> (w914:string)
                n1140 = local write "Insert flag"(TRUE ("Insert flag")) -> ()
                n1141 = call "CRYCalibration.vi"("O_Signal Type Old In"=w922, "I_Signal Type Old In"=w923, "Hardware In"=w914, "O_Calibrated Device Name Old In"=w916, "I_Calibrated Device Name Old In"=w917, "Calibration"=w915, "Proper VI No In"=w924) -> ("O_Calibrated Device Name Out"=w918:string[][], "I_Calibrated Device Name Out"=w919:string[][], "O_Signal Type Out"=w920:string[][], "I_Signal Type Out"=w921:string[][])  [unwired: 1 in]
                n1142 = property on="I_Signal Type Name" class="Arr (strict)"("Value"=w921) -> ()  [unwired: 2 in, 2 out]
                n1143 = property on="I_Calibrated Device Name" class="Arr (strict)"("Value"=w919) -> ()  [unwired: 2 in, 2 out]
                n1144 = property on="O_Calibrated Device Name" class="Arr (strict)"("Value"=w918) -> ()  [unwired: 2 in, 2 out]
                n1145 = property on="O_Signal Type Name" class="Arr (strict)"("Value"=w920) -> ()  [unwired: 2 in, 2 out]
              }
            }
          }
        }
      }
      frame 26 {
        n1146 = local write "stop"(TRUE ("stop")) -> ()
        n1147 = flat-sequence {
          frame #0 {
            n1148 = global read "CRYMainGlobal.vi" "Access Level"() -> (w926:enum16{"Engineer", "Technician", "Operator"})
            n1149 = case shown="\"Engineer\", Default" w926 {
              frame "Engineer", Default {
                n1150 = flat-sequence {
                  tunnel: [w934] -> w930
                  tunnel: [w933] -> w929
                  tunnel: [w932] -> w927
                  tunnel: [w939] -> w931
                  tunnel: w930 -> [w939]
                  tunnel: w929 -> [w938]
                  tunnel: [w937] -> w928
                  tunnel: w927 -> [w937]
                  tunnel: w931 -> [w955]
                  tunnel: w928 -> [w951]
                  frame #0 {
                    n1151 = local read "Calibration"() -> (w935:T1)
                    n1152 = call "CRYUpdate Calibration Date.vi"("Calibration In"=w935) -> ("Calibration Out"=w933:T1)  [unwired: 10 in]
                    n1153 = call "CRYFlatten Calibration 2D.vi"("Calibration All Cluster"=w933) -> ("Calibration flattened"=w934:string)  [unwired: 10 in]
                    n1154 = local write "Calibration"(w933) -> ()
                    n1155 = global read "CRYProject Editor Global.vi" "Calibration Step"() -> (w936:T6)
                    n1156 = Bundle By Name(cluster=w936, "Seq setup flattened"=w934) -> (w932:T6)
                  }
                  frame #1 {
                    n1157 = local read "Proper VI No"() -> (w950:i32)
                    n1158 = local read "Hardware In"() -> (w941:string)
                    n1159 = property on="I_Calibrated Device Name" class="Arr (strict)"() -> ("Value"=w947:string[][])  [unwired: 2 in, 2 out]
                    n1160 = property on="O_Calibrated Device Name" class="Arr (strict)"() -> ("Value"=w946:string[][])  [unwired: 2 in, 2 out]
                    n1161 = property on="O_Signal Type Name" class="Arr (strict)"() -> ("Value"=w948:string[][])  [unwired: 2 in, 2 out]
                    n1162 = property on="I_Signal Type Name" class="Arr (strict)"() -> ("Value"=w949:string[][])  [unwired: 2 in, 2 out]
                    n1163 = call "CRYCalibration.vi"("O_Signal Type Old In"=w948, "Apply?"=TRUE, "I_Signal Type Old In"=w949, "Hardware In"=w941, "O_Calibrated Device Name Old In"=w946, "I_Calibrated Device Name Old In"=w947, "Calibration"=w938, "Proper VI No In"=w950) -> ("O_Calibrated Device Name Out"=w942:string[][], "I_Calibrated Device Name Out"=w943:string[][], "O_Signal Type Out"=w944:string[][], "I_Signal Type Out"=w945:string[][])
                    n1164 = property on="I_Signal Type Name" class="Arr (strict)"("Value"=w945) -> ()  [unwired: 2 in, 2 out]
                    n1165 = property on="O_Signal Type Name" class="Arr (strict)"("Value"=w944) -> ()  [unwired: 2 in, 2 out]
                    n1166 = property on="I_Calibrated Device Name" class="Arr (strict)"("Value"=w943) -> ()  [unwired: 2 in, 2 out]
                    n1167 = property on="O_Calibrated Device Name" class="Arr (strict)"("Value"=w942) -> ()  [unwired: 2 in, 2 out]
                  }
                  frame #2 {
                    w956 = "Calibration" ("Step File Name")
                    n1168 = global read "CRYMainGlobal.vi" "Calibration path"() -> (w953:path)
                    n1169 = global write "CRYProject Editor Global.vi" "Calibration Step"(w951) -> ()
                    n1170 = Build Path(base path=w953, name or relative path="Calibration Default.cal") -> (appended path=w954:path)
                    n1171 = call "CRYStep Write.vi"("Category Name"=w956, "All/Name/Write(0,1,2)?"=u8 2, "Step File Path"=w954, "Step flattened"=w955, "Step File Name"=w956) -> ()  [unwired: 4 in, 3 out]
                  }
                }
              }
              frame "Operator" {
                n1172 = call "CRYGet Error Message.vi"("Kind"="Step Setup") -> ("Window Title"=w961:string)  [unwired: 5 in, 5 out]
                n1173 = call "CRYGet Access Level Message.vi"("sAction"="OK") -> ("Multibyte string"=w959:string)  [unwired: 10 in]
                n1174 = call "CRYMessage Dialog.vi"("Window Title"=w961, "YesNoCancel"=T8."OK", "Message Content"=w959) -> ()  [unwired: 7 in, 2 out]
              }
            }
          }
          frame #1 {
            n1175 = local write "SaveCalibration"(FALSE ("OK")) -> ()
          }
        }
      }
      frame 27 {
        n1176 = local write "Cancel"(FALSE ("Cancel")) -> ()
        n1177 = local write "stop"(TRUE ("stop")) -> ()
      }
      frame Default {
      }
    }
  }
  n1178 = flat-sequence {
    tunnel: w1 -> [_]
    frame #0 {
      n1179 = control-ref of="This VI"() -> (w1472:refnum<vi>)
      n1180 = call "CRYWork Before Step Close.vi"("StepVI Ref"=w1472) -> ()  [unwired: 11 in]
    }
    frame #1 {
      n1181 = local write "EndFlag"(TRUE ("EndFlag")) -> ()
    }
  }
